vi "01_ui_main_loop.vi"() -> ()   [LabVIEW 2025]
uses:
  0417e9bc-26c0-40a3-857c-749a2451377f.vi
  040e489e-a473-4f93-bd06-0afa5652ce70.vi
  c6e3c1e2-0994-45fa-bff3-5cd5cb70e039.vi
  0bc7f4c2-ffb1-4822-9f64-357063f019c3.vi
  8b609e5e-a51d-4c52-8c18-d6a58a5b9e80.vi
  43d63275-3364-44ab-a9c8-6f7e055a0a8e.vi
  75836779-3642-44ab-91a1-288c14d5bff7.vi
  f856a27e-8979-4d67-ac65-7e3e0066168f.vi
  f6c46c24-e81c-4bed-970f-882e3bbfa33a.vi
  674b8dbc-10ac-464c-a410-8119d69976f5.vi
  efe7b7fb-95db-4648-be1d-36dd24965d64.vi
  a7921508-b016-4ad4-9c73-64ec30acdca8.vi
  2bf2835e-c011-4d5e-a055-403be64c671f.vi
  <vilib>/Utility/config.llb/Read Key (String).vi
  <vilib>/Utility/config.llb/Read Key (U32).vi
  <vilib>/Utility/config.llb/Read Key (Boolean).vi
  <vilib>/Utility/config.llb/Write Key (String).vi
  <vilib>/Utility/config.llb/Write Key (U32).vi
  <vilib>/Utility/config.llb/Write Key (Boolean).vi
  <vilib>/Utility/config.llb/NI_LVConfig.lvlib
panel:
  in  "color_picker_cursor_2":u32(colorbox)=16756736
  in  "color_picker_cursor_1":u32(colorbox)=11927752
  in  "sva_del_cal_file":bool
  in  "sva_cal_file":string(combo)
  in  "button_tcp_load_cal":bool caption="Connect"
  in  "button_tcp_smith_mode":bool caption="Connect"
  in  "button_tcp_s21_mode":bool caption="Connect"
  in  "button_tcp_s11_mode":bool caption="Connect"
  in  "button_tcp_vna_mode":bool caption="Connect"
  in  "show_plot_window":bool
  in  "button_save_s2p":bool caption="Save *.s2p"
  in  "button_tcp_connect":bool caption="Connect"
  in  "sva_port":u16=5025 caption="Port"
  in  "sva_ip":string="192.168.2.29" caption="IP"
  in  "stop":bool
  in  "button_auto_sweep":bool caption="Auto Sweep"
  in  "sweep_points":dbl caption="Points" min=0.0 step=1.0 format="%#_6f"
  in  "sweep_stop":dbl caption="Stop Frequency" min=0.0 step=1.0 format="%#_6f"
  in  "sweep_start":dbl caption="Start Frequency" min=0.0 step=1.0 format="%#_6f"
  in  "selector_serial_port":refnum<visa-resource-name>="COM1" caption="COM-Port"
  out "led_serial_connected":bool caption="Connected"
  in  "button_serial_connect":bool caption="Connect"
  in  "button_single_sweep":bool caption="Single Sweep"
  out "plot_smith_legend_curs_r":dbl caption="Cursor - R"
  out "plot_smith_legend_phase":dbl caption="Phase"
  out "plot_smith_legend_freq":string caption="Frequency"
  out "plot_smith_legend_jx":dbl caption="jX"
  out "plot_smith_legend_r":dbl caption="R"
  out "plot_smith":picture caption="Smith"
  out "filename":string caption="Recent File"
  in  "button_save_s1p":bool caption="Save *.s1p"
  in  "button_load_csv":bool caption="Load *.s1p 2"
  in  "button_load_sxp":bool caption="Load *.sxp"
  in  "show_smith_window":bool
  out "min_vswr_idx":i32
  in  "set_min_vswr_c2":bool
  in  "set_min_vswr_c1":bool
  out "min_vswr_freq":string caption="@ Frequency"
  out "min_vswr":dbl caption="Min. VSWR"
  out "min_frequency":string caption="Min. Frequency"
  out "points":dbl caption="Points"
  out "max_frequency":string caption="Max. Frequency"
  out "plot_smith_legend_curs_x":dbl caption="Cursor - jX"
  out "cursor_cp_1_prefix":string
  out "cursor_lp_1_prefix":string
  out "cursor_cs_1_prefix":string
  out "cursor_ls_1_prefix":string
  out "cursor_cp_2_prefix":string
  out "cursor_lp_2_prefix":string
  out "cursor_cs_2_prefix":string
  in  "lc_scale_settings":enum32{"autoscale", "fancy_scale", "zero_scale"}(radio)=enum."zero_scale"
  out "cursor_ls_2_prefix":string
  out "cursor_cp_2":dbl format="%#_6f"
  in  "color_picker_cp":u32(colorbox)=14468608
  out "cursor_cp_1":dbl format="%#_6f"
  in  "enable_plot_cp":bool=TRUE caption="S11 - Imaginary"
  out "cursor_lp_2":dbl format="%#_6f"
  in  "color_picker_lp":u32(colorbox)=39219
  out "cursor_lp_1":dbl format="%#_6f"
  in  "enable_plot_lp":bool caption="S11 - Imaginary"
  out "cursor_cs_2":dbl format="%#_6f"
  out "cursor_ls_2":dbl format="%#_6f"
  out "cursor_lc_freq_2":string caption="Frequenz"
  out "cursor_lc_wavel_2":dbl caption="Frequenz"
  out "cursor_lc_wavel_1":dbl caption="Frequenz"
  in  "color_picker_cs":u32(colorbox)=14423100
  in  "color_picker_ls":u32(colorbox)=26316
  out "cursor_lc_freq_1":string caption="Frequenz"
  out "cursor_cs_1":dbl format="%#_6f"
  out "cursor_ls_1":dbl format="%#_6f"
  in  "enable_plot_cs":bool caption="S11 - Imaginary"
  in  "enable_plot_ls":bool=TRUE caption="S11 - Real"
  out "plot_lc":cluster{"array type (2D Dbl)":dbl[], dbl[]}[](graph) caption="L+C (Serial) / Lp+Cp (Parallel)"
  out "cursor_z_2":dbl format="%#_6f"
  in  "color_picker_z":u32(colorbox)=13314815
  out "cursor_z_1":dbl format="%#_6f"
  in  "enable_plot_z":bool=TRUE caption="S11 - Imaginary"
  out "cursor_jxp_2":dbl format="%#_6f"
  in  "color_picker_jxp":u32(colorbox)=14468608
  out "cursor_jxp_1":dbl format="%#_6f"
  in  "enable_plot_jxp":bool caption="S11 - Imaginary"
  out "cursor_rp_2":dbl format="%#_6f"
  in  "color_picker_rp":u32(colorbox)=39219
  out "cursor_rp_1":dbl format="%#_6f"
  in  "enable_plot_rp":bool caption="S11 - Imaginary"
  out "cursor_jx_2":dbl format="%#_6f"
  out "cursor_r_2":dbl format="%#_6f"
  out "cursor_imag_2":dbl format="%#_6f"
  out "cursor_real_2":dbl format="%#_6f"
  out "cursor_r_jx_freq_2":string caption="Frequenz"
  out "cursor_r_jx_wavel_2":dbl caption="Frequenz"
  out "cursor_r_jx_wavel_1":dbl caption="Frequenz"
  out "cursor_real_imag_freq_2":string caption="Frequenz"
  out "cursor_real_imag_wavel_2":dbl caption="Frequenz"
  out "cursor_real_imag_wavel_1":dbl caption="Frequenz"
  out "cursor_log_phase_wavel_2":dbl caption="Frequenz"
  out "cursor_log_phase_wavel_1":dbl caption="Frequenz"
  in  "cursor_mode":bool=TRUE caption="Cursor Mode"
  out "cursor_vswr_2":dbl format="%#_6f"
  in  "color_picker_vswr":u32(colorbox)=39219
  out "cursor_vswr_1":dbl format="%#_6f"
  in  "enable_plot_vswr":bool=TRUE caption="S11 - VSWR"
  out "cursor_log_phase_freq_2":string caption="Frequenz"
  out "cursor_phase_2":dbl format="%#_6f"
  out "cursor_logmag_2":dbl format="%#_6f"
  in  "color_picker_jx":u32(colorbox)=14423100
  in  "color_picker_r":u32(colorbox)=26316
  out "cursor_r_jx_freq_1":string caption="Frequenz"
  out "cursor_jx_1":dbl format="%#_6f"
  out "cursor_r_1":dbl format="%#_6f"
  in  "enable_plot_jx":bool=TRUE caption="S11 - Imaginary"
  in  "enable_plot_r":bool=TRUE caption="S11 - Real"
  in  "color_picker_imag":u32(colorbox)=14423100
  in  "color_picker_real":u32(colorbox)=26316
  out "cursor_real_imag_freq_1":string caption="Frequenz"
  out "cursor_imag_1":dbl format="%#_6f"
  out "cursor_real_1":dbl format="%#_6f"
  in  "enable_plot_imag":bool=TRUE caption="S11 - Imaginary"
  in  "enable_plot_real":bool=TRUE caption="S11 - Real"
  out "plot_real_imag":cluster{"array type (2D Dbl)":dbl[], dbl[]}[](graph) caption="Real / Imaginary"
  in  "color_picker_phase":u32(colorbox)=14423100
  in  "color_picker_logmag":u32(colorbox)=26316
  out "cursor_log_phase_freq_1":string caption="Frequenz"
  out "cursor_phase_1":dbl format="%#_6f"
  out "cursor_logmag_1":dbl format="%#_6f"
  in  "rx_scale_settings":enum32{"autoscale", "fancy_scale"}(radio)=enum."fancy_scale"
  in  "enable_plot_phase":bool=TRUE caption="S11 - Phase"
  in  "enable_plot_logmag":bool=TRUE caption="S11 - Logmag"
  out "plot_rjx":cluster{"array type (2D Dbl)":dbl[], dbl[]}[](graph) caption="R+jX (Serial) / Rp+jXp (Parallel) / Z"
  out "plot_log_phase_vswr":cluster{"array type (2D Dbl)":dbl[], dbl[]}[](graph) caption="Logmag / Phase / VSWR"
  # "LabVNA - VNA/S-Parameter Software"
  # "by Robin Tönniges (DC7RT)"
  # "Hz"
  # "NanoVNA"
  # "Siglent SVA"
  # "Sweep"
  # "Trace Data"
  # "Load/Save"
  # "Cursor 1"
  # "Cursor 2"
  # "Frequency"
  # "Hz"
  # "Hz"
  # "Wavelength"
  # "m"
  # "m"
  # "Frequency"
  # "Hz"
  # "Hz"
  # "Wavelength"
  # "m"
  # "m"
  # "Hz"
  # "Frequency"
  # "Hz"
  # "Wavelength"
  # "m"
  # "m"
  # "Frequency [MHz]"
  # "Hz"
  # "Frequency"
  # "Hz"
  # "Wavelength"
  # "m"
  # "m"
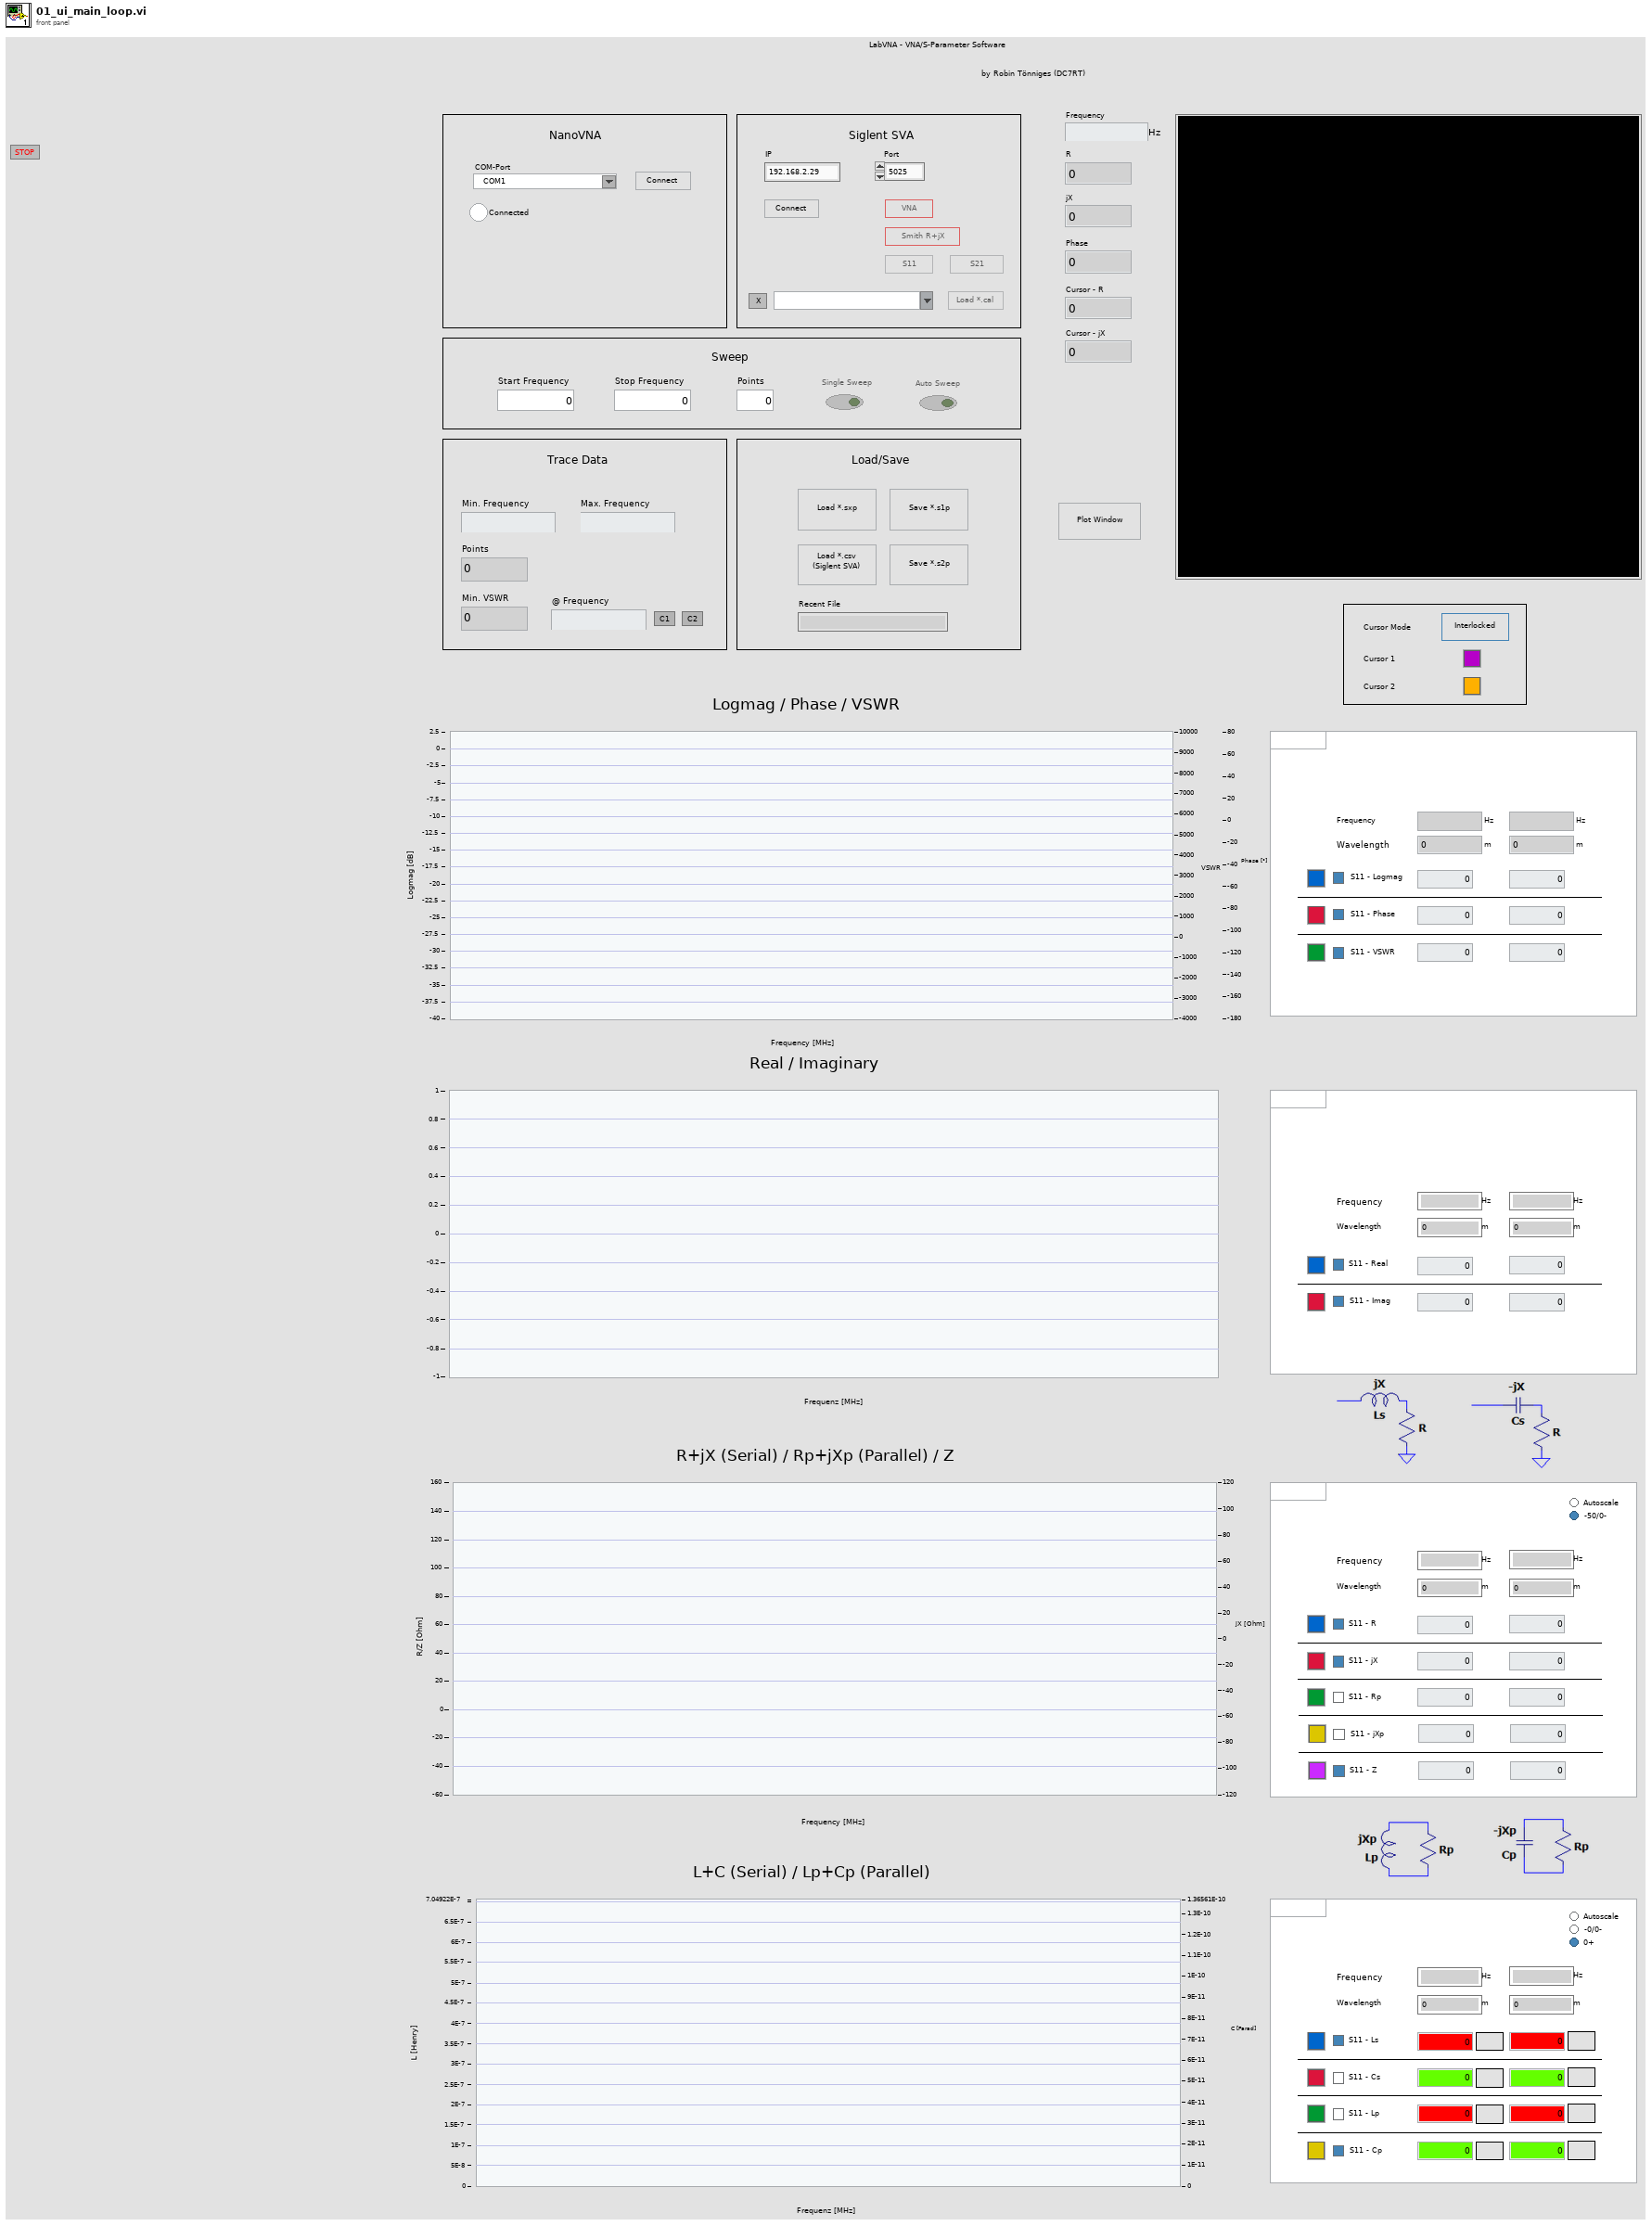
[diagram p1: front panel]
types:
  T1 = cluster{"button_serial_connect":bool, "button_auto_sweep":bool, "button_tcp_connect":bool}
  T2 = cluster{"button_load_sxp":bool, "button_load_csv":bool, "button_save_s1p":bool, "button_save_s2p":bool, "button_single_sweep":bool, "tcp_load_cal":bool}
  T3 = enum8{"Enabled", "Disabled", "Disabled and Grayed Out"}
  T4 = enum32{"Invalid", "Standard", "Closed", "Hidden", "Minimized", "Maximized"}
  T5 = cluster{"left":dbl, "top":dbl, "right":dbl, "bottom":dbl}
  T6 = cluster{"x":cluster{"a":dbl, "b":dbl, "log?":bool}, "y":cluster{"a":dbl, "b":dbl, "log?":bool}}
  T7 = typedef "NI_LVConfig.lvlib/Config Data RefNum.ctl" = refnum<k1>
  T8 = cluster{"button_load_sxp":bool, "button_load_csv":bool, "button_save_s1p":bool, "button_save_s2p":bool, "button_single_sweep":bool, "button_tcp_load_cal":bool}
  T9 = cluster{"mode":string, "s11_s21":string, "graph":string, "freq_range":cluster{"start_freq":string, "stop_freq":string}, "points":string}
  T10 = typedef "LVCursorListTypeDef.ctl" = cluster{"Name":string, "Color":u32, "Style":u8, "Point Style":u8, "Name Visible":bool, "Allow Drag":bool, "Cursor Mode":u32, "Plot":i32, "Index":i32, "Position":cluster{"X":dbl, "Y":dbl}, "X Scale":u32, "Y Scale":u32, "Watch Plots":i32[], "Watch All Plots":bool, "Plot Area":i32, "Label Offset":cluster{"X":dbl, "Y":dbl}}[]
  T11 = typedef "LVPoint32TypeDef.ctl" = cluster{"Horizontal":i32, "Vertical":i32}
  T12 = cluster{"frequency":dbl, "r":dbl, "jx":dbl, "phase":dbl}
  T13 = cluster{"cursor_data":dbl[], "frequency":string, "wavelength_m":dbl}
  T14 = cluster{"freq_array":dbl[], "data_array":dbl[]}[]
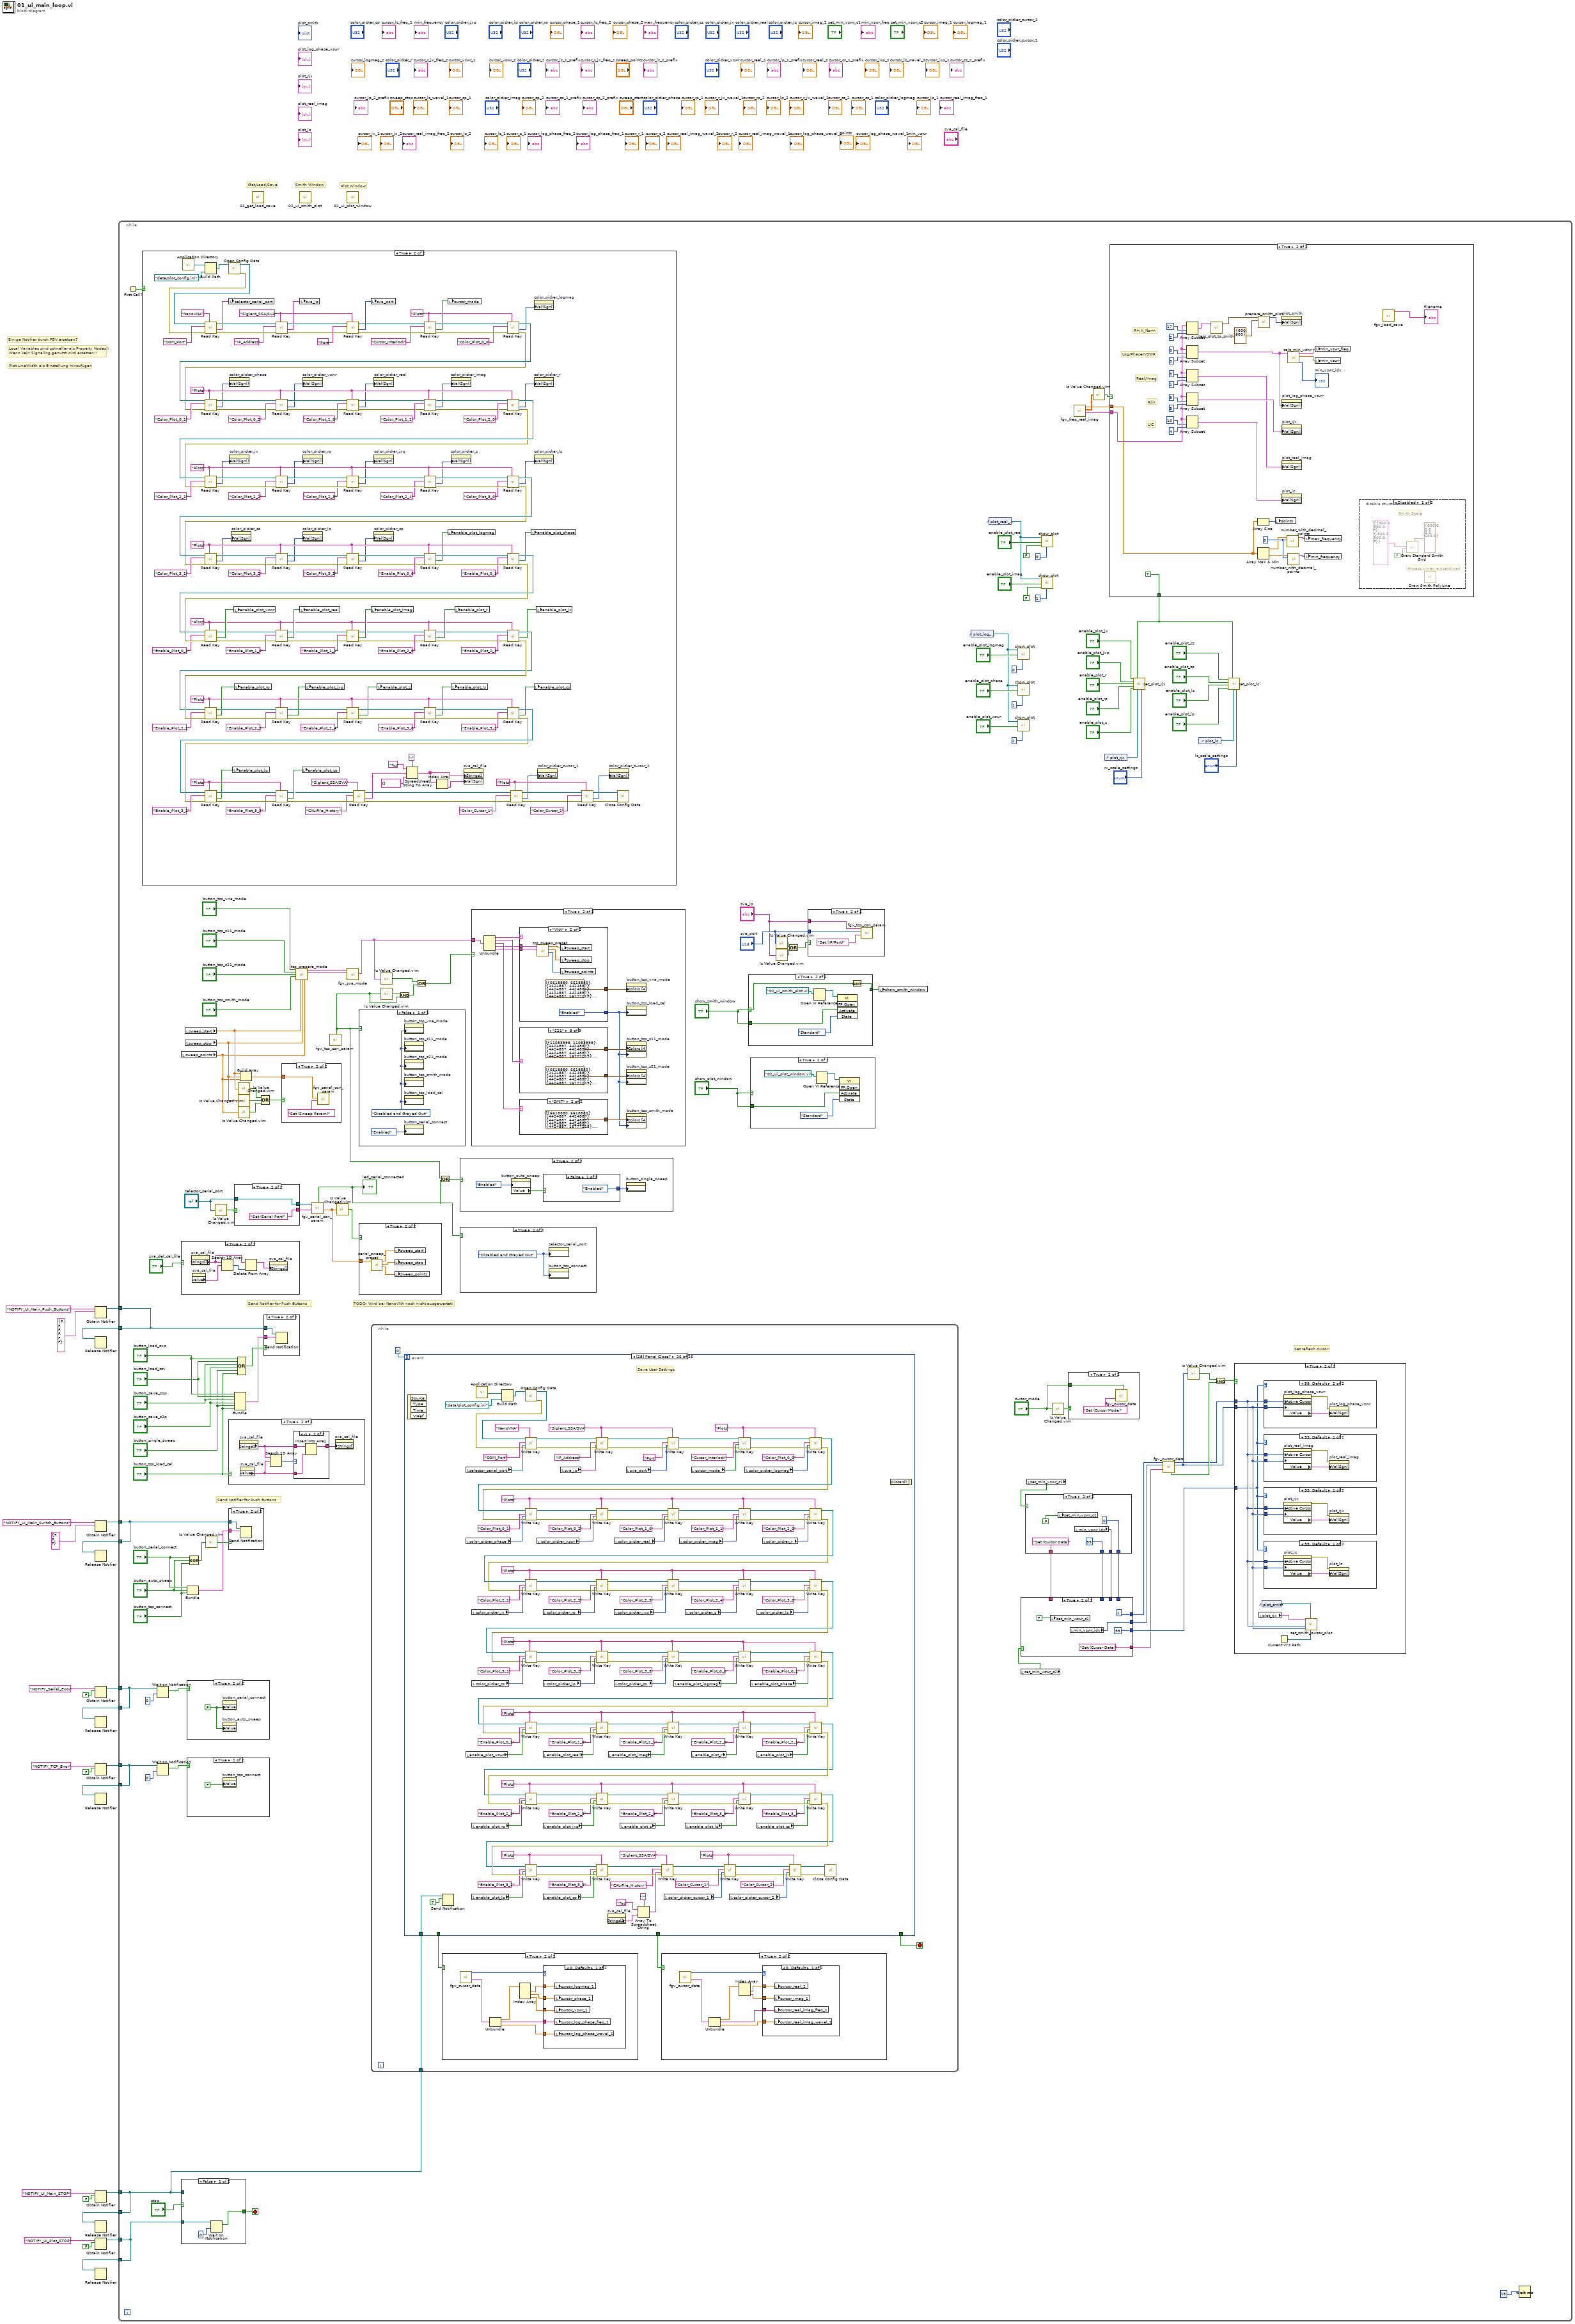
[diagram p0: block diagram]
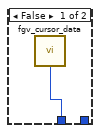
[diagram p9: hidden frame]
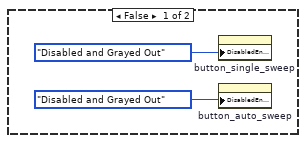
[diagram p11: hidden frame]
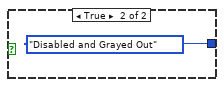
[diagram p12: hidden frame]
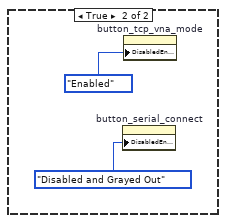
[diagram p16: hidden frame]
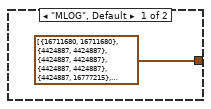
[diagram p18: hidden frame]
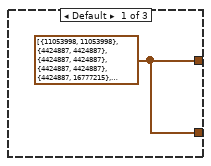
[diagram p19: hidden frame]
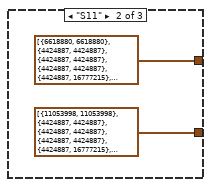
[diagram p20: hidden frame]
diagram:
  # "Plot LineWidth als Einstellung hinzufügen"
  # "Local Variables sind schneller als Property Nodes!!\nWenn kein Signaling genutzt wird ersetzen!!"
  # "Einige Notifier durch FGV ersetzen?"
  # "Plot Window"
  # "Get/Load/Save"
  # "Smith WIndow"
  n1 = Obtain Notifier(name (unnamed)="NOTIFY_UI_Main_Push_Buttons", notification data type=T2 {"button_load_sxp"=FALSE, "button_load_csv"=FALSE, "button_save_s1p"=FALSE, "button_save_s2p"=FALSE, "button_single_sweep"=FALSE, "tcp_load_cal"=FALSE} ("output cluster")) -> (notifier out=w23:refnum<notifier>)  [unwired: 2 in, 2 out]
  n2 = Obtain Notifier(name (unnamed)="NOTIFY_UI_Main_Switch_Buttons", notification data type=T1 {"button_serial_connect"=FALSE, "button_auto_sweep"=FALSE, "button_tcp_connect"=FALSE} ("output cluster")) -> (notifier out=w12:refnum<notifier>)  [unwired: 2 in, 2 out]
  n3 = Obtain Notifier(name (unnamed)="NOTIFY_Serial_Error", notification data type=FALSE) -> (notifier out=w15:refnum<notifier>)  [unwired: 2 in, 2 out]
  n4 = Obtain Notifier(name (unnamed)="NOTIFY_TCP_Error", notification data type=FALSE) -> (notifier out=w3:refnum<notifier>)  [unwired: 2 in, 2 out]
  n5 = Obtain Notifier(name (unnamed)="NOTIFY_UI_Main_STOP", notification data type=FALSE) -> (notifier out=w20:refnum<notifier>)  [unwired: 2 in, 2 out]
  n6 = Obtain Notifier(name (unnamed)="NOTIFY_UI_Plot_STOP", notification data type=FALSE) -> (notifier out=w6:refnum<notifier>)  [unwired: 2 in, 2 out]
  n7 = while {
    tunnel: w23 -> [w107]
    tunnel: [w107] -> w22
    tunnel: w20 -> [w84]
    tunnel: [w84] -> w21
    tunnel: w15 -> [w99]
    tunnel: [w99] -> w14
    tunnel: w12 -> [w96]
    tunnel: [w96] -> w13
    tunnel: [w73] -> w7
    tunnel: w6 -> [w73]
    tunnel: w3 -> [w66]
    tunnel: [w66] -> w4
    stop <- w100 stop-if-true
    # "Set refresh cursor"
    # "TODO: Wird bei NanoVNA noch nicht ausgewertet!"
    # "Send Notifier for Push Buttons"
    # "Send Notifier for Push Buttons"
    n8 = First Call?() -> (First Call?: T/F=w74:bool)
    n9 = case shown="True" w74 {
      frame False {
      }
      frame True {
        w251 = "Plots" ("section")
        w281 = "Plots" ("section")
        w272 = "Plots" ("section")
        w302 = "Plots" ("section")
        w271 = "Plots" ("section")
        w355 = "Plots" ("section")
        w356 = "Plots" ("section")
        w369 = "Plots" ("section")
        w370 = "Siglent_SSA/SVA" ("section")
        n10 = call <vilib>:"Application Directory.vi"() -> ("Application Directory"=w266:path)
        n11 = Build Path(base path=w266, name or relative path=path "data/plot_config.ini") -> (appended path=w270:path)
        n12 = call <vilib>:"Open Config Data.vi"("configuration file path"=w270) -> ("error out"=w268:errorcluster, "refnum"=w267:T7)  [unwired: 8 in, 1 out]
        n13 = call-poly <vilib>:"Read Key.vi"("section"="NanoVNA", "error in (no error)"=w268, "key"="COM_Port", "refnum"=w267) -> ("error out"=w386:errorcluster, "value"=w389:string, "refnum out"=w387:T7)  [unwired: 4 in, 1 out]
        n14 = local write "selector_serial_port"(w389) -> ()
        n15 = call-poly <vilib>:"Read Key.vi"("section"=w370, "error in (no error)"=w386, "key"="IP_Address", "refnum"=w387) -> ("error out"=w382:errorcluster, "value"=w385:string, "refnum out"=w383:T7)  [unwired: 4 in, 1 out]
        n16 = local write "sva_ip"(w385) -> ()
        n17 = call-poly <vilib>:"Read Key.vi"("section"=w370, "error in (no error)"=w382, "key"="Port", "refnum"=w383) -> ("error out"=w378:errorcluster, "value"=w381:u32, "refnum out"=w379:T7)  [unwired: 4 in, 1 out]
        n18 = local write "sva_port"(w381) -> ()
        n19 = call-poly <vilib>:"Read Key.vi"("section"=w369, "error in (no error)"=w378, "key"="Cursor_Interlock", "refnum"=w379) -> ("error out"=w374:errorcluster, "value"=w377:bool, "refnum out"=w375:T7)  [unwired: 4 in, 1 out]
        n20 = local write "cursor_mode"(w377) -> ()
        n21 = call-poly <vilib>:"Read Key.vi"("section"=w369, "error in (no error)"=w374, "key"="Color_Plot_0_0", "refnum"=w375) -> ("error out"=w371:errorcluster, "value"=w246:u32, "refnum out"=w372:T7)  [unwired: 4 in, 1 out]
        n22 = call-poly <vilib>:"Read Key.vi"("section"=w356, "error in (no error)"=w371, "key"="Color_Plot_0_1", "refnum"=w372) -> ("error out"=w366:errorcluster, "value"=w245:u32, "refnum out"=w367:T7)  [unwired: 4 in, 1 out]
        n23 = property on="color_picker_phase" class="ColBox"("Val(Sgnl)"=w245) -> ()  [unwired: 2 in, 2 out]
        n24 = call-poly <vilib>:"Read Key.vi"("section"=w356, "error in (no error)"=w366, "key"="Color_Plot_0_2", "refnum"=w367) -> ("error out"=w363:errorcluster, "value"=w244:u32, "refnum out"=w364:T7)  [unwired: 4 in, 1 out]
        n25 = property on="color_picker_vswr" class="ColBox"("Val(Sgnl)"=w244) -> ()  [unwired: 2 in, 2 out]
        n26 = call-poly <vilib>:"Read Key.vi"("section"=w356, "error in (no error)"=w363, "key"="Color_Plot_1_0", "refnum"=w364) -> ("error out"=w360:errorcluster, "value"=w243:u32, "refnum out"=w361:T7)  [unwired: 4 in, 1 out]
        n27 = property on="color_picker_real" class="ColBox"("Val(Sgnl)"=w243) -> ()  [unwired: 2 in, 2 out]
        n28 = call-poly <vilib>:"Read Key.vi"("section"=w356, "error in (no error)"=w360, "key"="Color_Plot_1_1", "refnum"=w361) -> ("error out"=w357:errorcluster, "value"=w242:u32, "refnum out"=w358:T7)  [unwired: 4 in, 1 out]
        n29 = property on="color_picker_imag" class="ColBox"("Val(Sgnl)"=w242) -> ()  [unwired: 2 in, 2 out]
        n30 = call-poly <vilib>:"Read Key.vi"("section"=w356, "error in (no error)"=w357, "key"="Color_Plot_2_0", "refnum"=w358) -> ("error out"=w340:errorcluster, "value"=w241:u32, "refnum out"=w341:T7)  [unwired: 4 in, 1 out]
        n31 = call-poly <vilib>:"Read Key.vi"("section"=w355, "error in (no error)"=w340, "key"="Color_Plot_2_1", "refnum"=w341) -> ("error out"=w345:errorcluster, "value"=w240:u32, "refnum out"=w344:T7)  [unwired: 4 in, 1 out]
        n32 = property on="color_picker_jx" class="ColBox"("Val(Sgnl)"=w240) -> ()  [unwired: 2 in, 2 out]
        n33 = call-poly <vilib>:"Read Key.vi"("section"=w355, "error in (no error)"=w345, "key"="Color_Plot_2_2", "refnum"=w344) -> ("error out"=w348:errorcluster, "value"=w239:u32, "refnum out"=w347:T7)  [unwired: 4 in, 1 out]
        n34 = property on="color_picker_rp" class="ColBox"("Val(Sgnl)"=w239) -> ()  [unwired: 2 in, 2 out]
        n35 = call-poly <vilib>:"Read Key.vi"("section"=w355, "error in (no error)"=w348, "key"="Color_Plot_2_3", "refnum"=w347) -> ("error out"=w351:errorcluster, "value"=w238:u32, "refnum out"=w350:T7)  [unwired: 4 in, 1 out]
        n36 = property on="color_picker_jxp" class="ColBox"("Val(Sgnl)"=w238) -> ()  [unwired: 2 in, 2 out]
        n37 = call-poly <vilib>:"Read Key.vi"("section"=w355, "error in (no error)"=w351, "key"="Color_Plot_2_4", "refnum"=w350) -> ("error out"=w354:errorcluster, "value"=w237:u32, "refnum out"=w353:T7)  [unwired: 4 in, 1 out]
        n38 = property on="color_picker_z" class="ColBox"("Val(Sgnl)"=w237) -> ()  [unwired: 2 in, 2 out]
        n39 = call-poly <vilib>:"Read Key.vi"("section"=w355, "error in (no error)"=w354, "key"="Color_Plot_3_0", "refnum"=w353) -> ("error out"=w331:errorcluster, "value"=w236:u32, "refnum out"=w332:T7)  [unwired: 4 in, 1 out]
        n40 = call-poly <vilib>:"Read Key.vi"("section"=w271, "error in (no error)"=w331, "key"="Color_Plot_3_1", "refnum"=w332) -> ("error out"=w336:errorcluster, "value"=w235:u32, "refnum out"=w337:T7)  [unwired: 4 in, 1 out]
        n41 = property on="color_picker_cs" class="ColBox"("Val(Sgnl)"=w235) -> ()  [unwired: 2 in, 2 out]
        n42 = call-poly <vilib>:"Read Key.vi"("section"=w271, "error in (no error)"=w336, "key"="Color_Plot_3_2", "refnum"=w337) -> ("error out"=w333:errorcluster, "value"=w234:u32, "refnum out"=w334:T7)  [unwired: 4 in, 1 out]
        n43 = property on="color_picker_lp" class="ColBox"("Val(Sgnl)"=w234) -> ()  [unwired: 2 in, 2 out]
        n44 = call-poly <vilib>:"Read Key.vi"("section"=w271, "error in (no error)"=w333, "key"="Color_Plot_3_3", "refnum"=w334) -> ("error out"=w295:errorcluster, "value"=w233:u32, "refnum out"=w294:T7)  [unwired: 4 in, 1 out]
        n45 = property on="color_picker_cp" class="ColBox"("Val(Sgnl)"=w233) -> ()  [unwired: 2 in, 2 out]
        n46 = call-poly <vilib>:"Read Key.vi"("section"=w271, "error in (no error)"=w295, "key"="Enable_Plot_0_0", "refnum"=w294) -> ("error out"=w300:errorcluster, "value"=w297:bool, "refnum out"=w299:T7)  [unwired: 4 in, 1 out]
        n47 = local write "enable_plot_logmag"(w297) -> ()
        n48 = call-poly <vilib>:"Read Key.vi"("section"=w271, "error in (no error)"=w300, "key"="Enable_Plot_0_1", "refnum"=w299) -> ("error out"=w322:errorcluster, "value"=w301:bool, "refnum out"=w321:T7)  [unwired: 4 in, 1 out]
        n49 = call-poly <vilib>:"Read Key.vi"("section"=w302, "error in (no error)"=w322, "key"="Enable_Plot_0_2", "refnum"=w321) -> ("error out"=w315:errorcluster, "value"=w319:bool, "refnum out"=w316:T7)  [unwired: 4 in, 1 out]
        n50 = local write "enable_plot_vswr"(w319) -> ()
        n51 = call-poly <vilib>:"Read Key.vi"("section"=w302, "error in (no error)"=w315, "key"="Enable_Plot_1_0", "refnum"=w316) -> ("error out"=w311:errorcluster, "value"=w318:bool, "refnum out"=w312:T7)  [unwired: 4 in, 1 out]
        n52 = local write "enable_plot_real"(w318) -> ()
        n53 = call-poly <vilib>:"Read Key.vi"("section"=w302, "error in (no error)"=w311, "key"="Enable_Plot_1_1", "refnum"=w312) -> ("error out"=w307:errorcluster, "value"=w313:bool, "refnum out"=w309:T7)  [unwired: 4 in, 1 out]
        n54 = local write "enable_plot_imag"(w313) -> ()
        n55 = call-poly <vilib>:"Read Key.vi"("section"=w302, "error in (no error)"=w307, "key"="Enable_Plot_2_0", "refnum"=w309) -> ("error out"=w304:errorcluster, "value"=w308:bool, "refnum out"=w305:T7)  [unwired: 4 in, 1 out]
        n56 = local write "enable_plot_r"(w308) -> ()
        n57 = call-poly <vilib>:"Read Key.vi"("section"=w302, "error in (no error)"=w304, "key"="Enable_Plot_2_1", "refnum"=w305) -> ("error out"=w330:errorcluster, "value"=w303:bool, "refnum out"=w329:T7)  [unwired: 4 in, 1 out]
        n58 = call-poly <vilib>:"Read Key.vi"("section"=w272, "error in (no error)"=w330, "key"="Enable_Plot_2_2", "refnum"=w329) -> ("error out"=w328:errorcluster, "value"=w324:bool, "refnum out"=w327:T7)  [unwired: 4 in, 1 out]
        n59 = local write "enable_plot_rp"(w324) -> ()
        n60 = call-poly <vilib>:"Read Key.vi"("section"=w272, "error in (no error)"=w328, "key"="Enable_Plot_2_3", "refnum"=w327) -> ("error out"=w283:errorcluster, "value"=w325:bool, "refnum out"=w282:T7)  [unwired: 4 in, 1 out]
        n61 = local write "enable_plot_jxp"(w325) -> ()
        n62 = call-poly <vilib>:"Read Key.vi"("section"=w272, "error in (no error)"=w283, "key"="Enable_Plot_2_4", "refnum"=w282) -> ("error out"=w289:errorcluster, "value"=w285:bool, "refnum out"=w287:T7)  [unwired: 4 in, 1 out]
        n63 = local write "enable_plot_z"(w285) -> ()
        n64 = call-poly <vilib>:"Read Key.vi"("section"=w272, "error in (no error)"=w289, "key"="Enable_Plot_3_0", "refnum"=w287) -> ("error out"=w292:errorcluster, "value"=w288:bool, "refnum out"=w291:T7)  [unwired: 4 in, 1 out]
        n65 = local write "enable_plot_ls"(w288) -> ()
        n66 = call-poly <vilib>:"Read Key.vi"("section"=w272, "error in (no error)"=w292, "key"="Enable_Plot_3_1", "refnum"=w291) -> ("error out"=w273:errorcluster, "value"=w293:bool, "refnum out"=w274:T7)  [unwired: 4 in, 1 out]
        n67 = call-poly <vilib>:"Read Key.vi"("section"=w281, "error in (no error)"=w273, "key"="Enable_Plot_3_2", "refnum"=w274) -> ("error out"=w280:errorcluster, "value"=w276:bool, "refnum out"=w279:T7)  [unwired: 4 in, 1 out]
        n68 = local write "enable_plot_lp"(w276) -> ()
        n69 = call-poly <vilib>:"Read Key.vi"("section"=w281, "error in (no error)"=w280, "key"="Enable_Plot_3_3", "refnum"=w279) -> ("error out"=w262:errorcluster, "value"=w277:bool, "refnum out"=w263:T7)  [unwired: 4 in, 1 out]
        n70 = local write "enable_plot_cp"(w277) -> ()
        n71 = call-poly <vilib>:"Read Key.vi"("section"="Siglent_SSA/SVA", "error in (no error)"=w262, "key"="CAL-File_History", "refnum"=w263) -> ("error out"=w253:errorcluster, "value"=w265:string, "refnum out"=w254:T7)  [unwired: 4 in, 1 out]
        n72 = Spreadsheet String To Array(delimiter (Tab)=";", format string="%s", spreadsheet string=w265, array type (2D Dbl)=string[] []) -> (array=w257:string[])
        n73 = Index Array(array=w257) -> (element=w256:string)  [unwired: 1 in]
        n74 = property on="sva_cal_file" class="CmbBox"("Strings[]"=w257, "Val(Sgnl)"=w256) -> ()  [unwired: 2 in, 2 out]
        n75 = call-poly <vilib>:"Read Key.vi"("section"=w251, "error in (no error)"=w253, "key"="Color_Cursor_1", "refnum"=w254) -> ("error out"=w247:errorcluster, "value"=w232:u32, "refnum out"=w248:T7)  [unwired: 4 in, 1 out]
        n76 = local write "enable_plot_phase"(w301) -> ()
        n77 = property on="color_picker_logmag" class="ColBox"("Val(Sgnl)"=w246) -> ()  [unwired: 2 in, 2 out]
        n78 = property on="color_picker_r" class="ColBox"("Val(Sgnl)"=w241) -> ()  [unwired: 2 in, 2 out]
        n79 = property on="color_picker_ls" class="ColBox"("Val(Sgnl)"=w236) -> ()  [unwired: 2 in, 2 out]
        n80 = local write "enable_plot_cs"(w293) -> ()
        n81 = local write "enable_plot_jx"(w303) -> ()
        n82 = property on="color_picker_cursor_1" class="ColBox"("Val(Sgnl)"=w232) -> ()  [unwired: 2 in, 2 out]
        n83 = call-poly <vilib>:"Read Key.vi"("section"=w251, "error in (no error)"=w247, "key"="Color_Cursor_2", "refnum"=w248) -> ("error out"=w249:errorcluster, "value"=w231:u32, "refnum out"=w250:T7)  [unwired: 4 in, 1 out]
        n84 = property on="color_picker_cursor_2" class="ColBox"("Val(Sgnl)"=w231) -> ()  [unwired: 2 in, 2 out]
        n85 = call <vilib>:"Close Config Data.vi"("error in (no error)"=w249, "refnum"=w250) -> ()  [unwired: 8 in, 2 out]
      }
    }
    n86 = Wait on Notification(notifier=w99, timeout in ms (-1)=0) -> (notification=w97:bool)  [unwired: 2 in, 3 out]
    n87 = Wait on Notification(notifier=w66, timeout in ms (-1)=0) -> (notification=w68:bool)  [unwired: 2 in, 3 out]
    n88 = case shown="True" "sva_del_cal_file" {
      frame False {
      }
      frame True {
        n89 = property on="sva_cal_file" class="CmbBox"() -> ("Strings[]"=w188:string[])  [unwired: 2 in, 2 out]
        n90 = property on="sva_cal_file" class="CmbBox"() -> ("Value"=w190:string)  [unwired: 2 in, 2 out]
        n91 = Search 1D Array(1D array=w188, element=w190) -> (index of element=w189:i32)  [unwired: 1 in]
        n92 = Delete From Array(array=w188, index=w189) -> (array with subset deleted=w187:string[])  [unwired: 1 in, 1 out]
        n93 = property on="sva_cal_file" class="CmbBox"("Strings[]"=w187) -> ()  [unwired: 2 in, 2 out]
      }
    }
    n94 = case shown="False" "stop" {
      selector: "stop" -> [_ w406]
      tunnel: w84 -> [_ w407]
      tunnel: [w403 FALSE] -> w100
      tunnel: w73 -> [w402 _]
      frame False {
        n95 = Wait on Notification(notifier=w402, timeout in ms (-1)=0) -> (notification=w403:bool)  [unwired: 2 in, 3 out]
      }
      frame True {
        n96 = Send Notification(notification=w406, notifier=w407) -> ()  [unwired: 1 in, 2 out]
      }
    }
    n97 = local read "sweep_points"() -> (w43:dbl)
    n98 = local read "sweep_start"() -> (w45:dbl)
    n99 = local read "sweep_stop"() -> (w44:dbl)
    n100 = Bundle("button_serial_connect"="button_serial_connect", "button_auto_sweep"="button_auto_sweep", "button_tcp_connect"="button_tcp_connect") -> (w69:T1)  [unwired: 1 in]
    n101 = case shown="True" w97 {
      frame False {
      }
      frame True {
        w401 = FALSE
        n102 = property on="button_serial_connect" class="Bool (strict)"("Value"=w401) -> ()  [unwired: 2 in, 2 out]
        n103 = property on="button_auto_sweep" class="Bool (strict)"("Value"=w401) -> ()  [unwired: 2 in, 2 out]
      }
    }
    n104 = case shown="True" w68 {
      frame False {
      }
      frame True {
        n105 = property on="button_tcp_connect" class="Bool (strict)"("Value"=FALSE) -> ()  [unwired: 2 in, 2 out]
      }
    }
    n106 = Compound Arithmetic op=XOR("button_serial_connect", "button_auto_sweep", "button_tcp_connect") -> (w91:bool)
    n107 = call "Is Value Changed.vim"("value"=w91) -> ("changed or first call?"=w92:bool)
    n108 = call "Is Value Changed.vim"("value"="selector_serial_port") -> ("changed or first call?"=w136:bool)
    n109 = case shown="True" "button_tcp_load_cal" {
      frame False {
      }
      frame True {
        n110 = property on="sva_cal_file" class="CmbBox"() -> ("Strings[]"=w193:string[])  [unwired: 2 in, 2 out]
        n111 = property on="sva_cal_file" class="CmbBox"() -> ("Value"=w192:string)  [unwired: 2 in, 2 out]
        n112 = Search 1D Array(1D array=w193, element=w192) -> (index of element=w194:i32)  [unwired: 1 in]
        n113 = case shown="-1" w194 {
          tunnel: w193 -> [w195 w198]
          tunnel: w192 -> [_ w197]
          tunnel: [w195 w196] -> w191
          frame 0, Default {
          }
          frame -1 {
            n114 = Insert Into Array(array=w198, new element=w197) -> (w196:string[])  [unwired: 1 in]
          }
        }
        n115 = property on="sva_cal_file" class="CmbBox"("Strings[]"=w191) -> ()  [unwired: 2 in, 2 out]
      }
    }
    n116 = case shown="True" w92 {
      tunnel: w96 -> [_ w400]
      tunnel: w69 -> [_ w399]
      frame False {
      }
      frame True {
        n117 = Send Notification(notification=w399, notifier=w400) -> ()  [unwired: 1 in, 2 out]
      }
    }
    n118 = case shown="True" w136 {
      tunnel: "selector_serial_port" -> [_ w417]
      tunnel: ["Get" ("mode") "Set (Serial Port)" ("mode")] -> w75
      tunnel: [_ w417] -> w76
      frame False {
      }
      frame True {
      }
    }
    n119 = Bundle("button_load_sxp"="button_load_sxp", "button_load_csv"="button_load_csv", "button_save_s1p"="button_save_s1p", "button_save_s2p"="button_save_s2p", "button_single_sweep"="button_single_sweep", "button_tcp_load_cal"="button_tcp_load_cal") -> (w79:T8)  [unwired: 1 in]
    n120 = Compound Arithmetic op=OR("button_load_sxp", "button_load_csv", "button_save_s1p", "button_save_s2p", "button_single_sweep", "button_tcp_load_cal") -> (w102:bool)
    n121 = call "Is Value Changed.vim"("value"=w45) -> ("changed or first call?"=w48:bool)
    n122 = call "Is Value Changed.vim"("value"=w44) -> ("changed or first call?"=w49:bool)
    n123 = call "Is Value Changed.vim"("value"=w43) -> ("changed or first call?"=w47:bool)
    n124 = Build Array(w45, w44, w43) -> (w42:dbl[])
    n125 = Compound Arithmetic op=OR(w48, w49, w47) -> (w46:bool)
    n126 = case shown="True" w102 {
      tunnel: w107 -> [_ w409]
      tunnel: w79 -> [_ w408]
      frame False {
      }
      frame True {
        n127 = Send Notification(notification=w408, notifier=w409) -> ()  [unwired: 1 in, 2 out]
      }
    }
    n128 = case shown="True" w46 {
      tunnel: w42 -> [_ w178]
      frame False {
      }
      frame True {
        n129 = call "fgv_serial_con_param.vi"("mode"="Set (Sweep Param)", "sweep_param_set"=w178) -> ()  [unwired: 5 in, 5 out]
      }
    }
    n130 = call "tcp_prepare_mode.vi"("button_tcp_vna_mode"="button_tcp_vna_mode", "button_tcp_s11_mode"="button_tcp_s11_mode", "button_tcp_s21_mode"="button_tcp_s21_mode", "button_tcp_smith_mode"="button_tcp_smith_mode", "sweep_start"=w45, "sweep_stop"=w44, "sweep_points"=w43) -> ("mode"=w58:string, "data_out"=w57:T9)  [unwired: 7 in]
    n131 = call "fgv_serial_con_param.vi"("mode"=w75, "serial_port_set"=w76) -> ("sweep_param_get"=w77:dbl[], "serial_conn_get"=w51:bool)  [unwired: 5 in, 3 out]
    "led_serial_connected" <- w51
    n132 = call "fgv_tcp_con_param.vi"() -> ("tcp_connected_get"=w50:bool)  [unwired: 8 in, 3 out]
    n133 = call "Is Value Changed.vim"("value"=w77) -> ("changed or first call?"=w134:bool)
    n134 = call "fgv_sva_mode.vi"("data_in"=w57, "mode"=w58) -> ("data_out"=w65:T9)  [unwired: 7 in, 2 out]
    n135 = case shown="False" w50 {
      frame False {
        w200 = T3."Disabled and Grayed Out" ("DisabledEnum")
        n136 = property on="button_tcp_vna_mode" class="Bool"("DisabledEnum"=w200) -> ()  [unwired: 2 in, 2 out]
        n137 = property on="button_tcp_s11_mode" class="Bool"("DisabledEnum"=w200) -> ()  [unwired: 2 in, 2 out]
        n138 = property on="button_tcp_s21_mode" class="Bool"("DisabledEnum"=w200) -> ()  [unwired: 2 in, 2 out]
        n139 = property on="button_tcp_smith_mode" class="Bool"("DisabledEnum"=w200) -> ()  [unwired: 2 in, 2 out]
        n140 = property on="button_tcp_load_cal" class="Bool"("DisabledEnum"=w200) -> ()  [unwired: 2 in, 2 out]
        n141 = property on="button_serial_connect" class="Bool (strict)"("DisabledEnum"=T3."Enabled" ("Disabled")) -> ()  [unwired: 2 in, 2 out]
      }
      frame True {
        n142 = property on="button_serial_connect" class="Bool (strict)"("DisabledEnum"=T3."Disabled and Grayed Out" ("Disabled")) -> ()  [unwired: 2 in, 2 out]
        n143 = property on="button_tcp_vna_mode" class="Bool"("DisabledEnum"=T3."Enabled") -> ()  [unwired: 2 in, 2 out]
      }
    }
    n144 = case shown="True" w134 {
      tunnel: w77 -> [_ w413]
      frame False {
      }
      frame True {
        n145 = call "serial_sweep_preset.vi"("sweep_data"=w413) -> ("sweep_points"=w412:dbl, "sweep_stop"=w411:dbl, "sweep_start"=w410:dbl)  [unwired: 8 in]
        n146 = local write "sweep_start"(w410) -> ()
        n147 = local write "sweep_stop"(w411) -> ()
        n148 = local write "sweep_points"(w412) -> ()
      }
    }
    n149 = while {
      tunnel: w84 -> [w428]
      stop <- w429 stop-if-true
      n150 = event shown="[25] Panel Close?" {
        selector: _ -> [_ _ _ _ _ _ _ _ _ _ _ _ _ _ _ _ _ _ _ _ _ _ _ _ _ _]
        dyn-events: _ -> [_ _ _ _ _ _ _ _ _ _ _ _ _ _ _ _ _ _ _ _ _ _ _ _ _ _]
        timeout: 0 -> [_ _ _ _ _ _ _ _ _ _ _ _ _ _ _ _ _ _ _ _ _ _ _ _ _ _]
        tunnel: [_ _ _ _ _ _ _ _ _ _ _ _ _ _ _ _ _ _ _ _ _ _ _ _ TRUE _] -> w429
        tunnel: w428 -> [_ _ _ _ _ _ _ _ _ _ _ _ _ _ _ _ _ _ _ _ _ _ _ _ _ w980]
        tunnel: [_ _ TRUE _ _ _ _ _ _ _ _ _ _ _ _ _ _ _ _ _ _ _ _ _ _ _] -> w427
        tunnel: [_ _ _ _ _ _ _ TRUE _ _ _ _ _ _ _ _ _ _ _ _ _ _ _ _ _ _] -> w426
        event "color_picker_cursor_1": Value Change {
          w472 = u32 0 ("Active Plot")
          n151 = event-data() -> ("NewVal"=w465:u32)  [unwired: 1 in, 5 out]
          n152 = Bundle("NewVal"=w465, "NewVal"=w465) -> (w466:cluster{"NewVal":u32, "NewVal":u32})  [unwired: 1 in]
          n153 = property on="plot_real_imag" class="XYGraph (strict)"("Active Cursor"=w472, "Cursor.Cursor Color"=w465) -> ()  [unwired: 2 in, 2 out]
          n154 = property on="plot_rjx" class="XYGraph (strict)"("Active Cursor"=w472, "Cursor.Cursor Color"=w465) -> ()  [unwired: 2 in, 2 out]
          n155 = property on="plot_lc" class="XYGraph (strict)"("Active Cursor"=w472, "Cursor.Cursor Color"=w465) -> ()  [unwired: 2 in, 2 out]
          n156 = property on="plot_log_phase_vswr" class="XYGraph (strict)"("Active Cursor"=w472, "Cursor.Cursor Color"=w465) -> ()  [unwired: 2 in, 2 out]
          n157 = property class="VI"() -> (error out=w470:errorcluster, "Front Panel"=w469:refnum<vi>)  [unwired: 2 in, 1 out]
          n158 = call "fgv_cursor_data.vi"("cursor_color_set"=w466, "mode"="Set (Cursor 0 Color)") -> ()  [unwired: 7 in, 7 out]
          n159 = property class="Pnl"(reference=w469, error in=w470) -> ("Decorations[]"=w468:refnum<vi>[])  [unwired: 2 out]
          n160 = Index Array(array=w468, index=0) -> (element=w471:refnum<vi>)
          n161 = property class="Decor"(reference=w471, "BG Color"=w465, "FG Color"=w465) -> ()  [unwired: 1 in, 2 out]
        }
        event "color_picker_cursor_2": Value Change {
          w481 = u32 1 ("Active Plot")
          n162 = event-data() -> ("NewVal"=w473:u32)  [unwired: 1 in, 5 out]
          n163 = Bundle("NewVal"=w473, "NewVal"=w473) -> (w475:cluster{"NewVal":u32, "NewVal":u32})  [unwired: 1 in]
          n164 = property on="plot_real_imag" class="XYGraph (strict)"("Active Cursor"=w481, "Cursor.Cursor Color"=w473) -> ()  [unwired: 2 in, 2 out]
          n165 = property on="plot_rjx" class="XYGraph (strict)"("Active Cursor"=w481, "Cursor.Cursor Color"=w473) -> ()  [unwired: 2 in, 2 out]
          n166 = property on="plot_lc" class="XYGraph (strict)"("Active Cursor"=w481, "Cursor.Cursor Color"=w473) -> ()  [unwired: 2 in, 2 out]
          n167 = property on="plot_log_phase_vswr" class="XYGraph (strict)"("Active Cursor"=w481, "Cursor.Cursor Color"=w473) -> ()  [unwired: 2 in, 2 out]
          n168 = property class="VI"() -> (error out=w479:errorcluster, "Front Panel"=w478:refnum<vi>)  [unwired: 2 in, 1 out]
          n169 = call "fgv_cursor_data.vi"("cursor_color_set"=w475, "mode"="Set (Cursor 1 Color)") -> ()  [unwired: 7 in, 7 out]
          n170 = property class="Pnl"(reference=w478, error in=w479) -> ("Decorations[]"=w477:refnum<vi>[])  [unwired: 2 out]
          n171 = Index Array(array=w477, index=1) -> (element=w480:refnum<vi>)
          n172 = property class="Decor"(reference=w480, "BG Color"=w473, "FG Color"=w473) -> ()  [unwired: 1 in, 2 out]
        }
        event "plot_log_phase_vswr": Cursor Move {
          # "Print Cursor Values for Logmag/Phase-Plot"
          n173 = event-data() -> ("CursIdx"=w486:i32, "CursRef"=w487:refnum<vi>)  [unwired: 1 in, 7 out]
          n174 = property on="Property Node" class="Curs"(reference=w487) -> ("Cursor Index"=w485:i32)  [unwired: 1 in, 2 out]
          n175 = local read "plot_log_phase_vswr"() -> (w483:cluster{"array type (2D Dbl)":dbl[], dbl[]}[])
          n176 = call "fgv_cursor_data.vi"("cursor_idx_set"=w486, "plot_data_set"=w483, "cursor_pos_set"=w485, "mode"="Set (Cursor Data)", "plot_id_set"=0) -> ()  [unwired: 4 in, 7 out]
        }
        event "plot_log_phase_vswr": Value Change {
          # "Print Cursor Values for Logmag/Phase-Plot"
          n177 = event-data() -> ("CtlRef"=w489:refnum<vi>, "NewVal"=w491:cluster{"array type (2D Dbl)":dbl[], dbl[]}[])  [unwired: 1 in, 4 out]
          n178 = property on="Property Node" class="XYGraph (strict)"(reference=w489) -> ("CrsrList"=w490:T10)  [unwired: 1 in, 2 out]
          n179 = Array Size(array=w490) -> (size(s)=w492:i32)
          n180 = for {
            N: w492 -> [_]
            tunnel: w490 -> [w506] mode=indexing
            tunnel: w491 -> [w500]
            i -> [w493]
            n181 = Unbundle By Name(w506) -> ("Index"=w494:i32)
            n182 = call "index_one_axis.vi"("x_index"=w494, "curve_sel"=0 ("x_index"), "graph_data"=w500) -> ("Y"=w497:dbl)  [unwired: 7 in, 1 out]
            n183 = call "index_one_axis.vi"("x_index"=w494, "curve_sel"=1 ("x_index"), "graph_data"=w500) -> ("Y"=w498:dbl)  [unwired: 7 in, 1 out]
            n184 = call "index_one_axis.vi"("x_index"=w494, "curve_sel"=2 ("x_index"), "graph_data"=w500) -> ("Y"=w499:dbl, "X"=w496:dbl)  [unwired: 7 in]
            n185 = call "number_with_decimal_points.vi"("Precision"=i16 0, "Double"=w496) -> ("String"=w505:string)  [unwired: 5 in]
            n186 = call "freq_to_wavelength.vi"("frequency_hz"=w496) -> ("wavelength_m"=w495:dbl)  [unwired: 10 in]
            n187 = case shown="0, Default" w493 {
              tunnel: w505 -> [w511 w516]
              tunnel: w498 -> [w510 w513]
              tunnel: w497 -> [w509 w514]
              tunnel: w499 -> [w508 w515]
              tunnel: w495 -> [w507 w512]
              frame 0, Default {
                n188 = local write "cursor_log_phase_freq_1"(w511) -> ()
                n189 = local write "cursor_log_phase_wavel_1"(w507) -> ()
                n190 = local write "cursor_logmag_1"(w509) -> ()
                n191 = local write "cursor_phase_1"(w510) -> ()
                n192 = local write "cursor_vswr_1"(w508) -> ()
              }
              frame 1 {
                n193 = local write "cursor_log_phase_freq_2"(w516) -> ()
                n194 = local write "cursor_log_phase_wavel_2"(w512) -> ()
                n195 = local write "cursor_phase_2"(w513) -> ()
                n196 = local write "cursor_vswr_2"(w515) -> ()
                n197 = local write "cursor_logmag_2"(w514) -> ()
              }
            }
          }
        }
        event "color_picker_logmag": Value Change {
          # "Change Plot Color Logmag/Phase-Plot [Logmag]"
          n198 = event-data() -> ("NewVal"=w517:u32)  [unwired: 1 in, 5 out]
          n199 = property on="plot_log_phase_vswr" class="XYGraph (strict)"("Active Plot"=u32 0, "Plot.Plot Color"=w517) -> ()  [unwired: 2 in, 2 out]
        }
        event "color_picker_phase": Value Change {
          # "Change Plot Color Logmag/Phase-Plot [Phase]"
          n200 = event-data() -> ("NewVal"=w519:u32)  [unwired: 1 in, 5 out]
          n201 = property on="plot_log_phase_vswr" class="XYGraph (strict)"("Active Plot"=u32 1, "Plot.Plot Color"=w519) -> ()  [unwired: 2 in, 2 out]
        }
        event "color_picker_vswr": Value Change {
          # "Change Plot Color Logmag/Phase-Plot [VSWR]"
          n202 = event-data() -> ("NewVal"=w521:u32)  [unwired: 1 in, 5 out]
          n203 = property on="plot_log_phase_vswr" class="XYGraph (strict)"("Active Plot"=u32 2, "Plot.Plot Color"=w521) -> ()  [unwired: 2 in, 2 out]
        }
        event "plot_real_imag": Cursor Move {
          # "Print Cursor Values for Real/Imag-Plot"
          n204 = event-data() -> ("CursIdx"=w526:i32, "CursRef"=w525:refnum<vi>)  [unwired: 1 in, 7 out]
          n205 = property on="Property Node" class="Curs"(reference=w525) -> ("Cursor Index"=w528:i32)  [unwired: 1 in, 2 out]
          n206 = local read "plot_real_imag"() -> (w524:cluster{"array type (2D Dbl)":dbl[], dbl[]}[])
          n207 = call "fgv_cursor_data.vi"("cursor_idx_set"=w526, "plot_data_set"=w524, "cursor_pos_set"=w528, "mode"="Set (Cursor Data)", "plot_id_set"=1) -> ()  [unwired: 4 in, 7 out]
        }
        event "plot_real_imag": Value Change {
          # "Print Cursor Values for Real/Imag-Plot"
          n208 = event-data() -> ("CtlRef"=w532:refnum<vi>, "NewVal"=w533:cluster{"array type (2D Dbl)":dbl[], dbl[]}[])  [unwired: 1 in, 4 out]
          n209 = property on="Property Node" class="XYGraph (strict)"(reference=w532) -> ("CrsrList"=w530:T10)  [unwired: 1 in, 2 out]
          n210 = Array Size(array=w530) -> (size(s)=w531:i32)
          n211 = for {
            N: w531 -> [_]
            tunnel: w533 -> [w542]
            tunnel: w530 -> [w538] mode=indexing
            i -> [w537]
            n212 = Unbundle By Name(w538) -> ("Index"=w536:i32)
            n213 = call "index_two_axes.vi"("x_index"=w536, "graph_data"=w542) -> ("Y2"=w540:dbl, "Y1"=w541:dbl, "X"=w534:dbl)  [unwired: 7 in]
            n214 = call "number_with_decimal_points.vi"("Precision"=i16 0, "Double"=w534) -> ("String"=w539:string)  [unwired: 5 in]
            n215 = call "freq_to_wavelength.vi"("frequency_hz"=w534) -> ("wavelength_m"=w535:dbl)  [unwired: 10 in]
            n216 = case shown="1" w537 {
              tunnel: w541 -> [w547 w548]
              tunnel: w540 -> [w546 w549]
              tunnel: w539 -> [w545 w550]
              tunnel: w535 -> [w544 w551]
              frame 0, Default {
                n217 = local write "cursor_real_1"(w547) -> ()
                n218 = local write "cursor_imag_1"(w546) -> ()
                n219 = local write "cursor_real_imag_freq_1"(w545) -> ()
                n220 = local write "cursor_real_imag_wavel_1"(w544) -> ()
              }
              frame 1 {
                n221 = local write "cursor_real_imag_freq_2"(w550) -> ()
                n222 = local write "cursor_real_imag_wavel_2"(w551) -> ()
                n223 = local write "cursor_real_2"(w548) -> ()
                n224 = local write "cursor_imag_2"(w549) -> ()
              }
            }
          }
        }
        event "color_picker_real": Value Change {
          n225 = event-data() -> ("NewVal"=w552:u32)  [unwired: 1 in, 5 out]
          n226 = property on="plot_real_imag" class="XYGraph (strict)"("Active Plot"=u32 0, "Plot.Plot Color"=w552) -> ()  [unwired: 2 in, 2 out]
        }
        event "color_picker_imag": Value Change {
          n227 = event-data() -> ("NewVal"=w554:u32)  [unwired: 1 in, 5 out]
          n228 = property on="plot_real_imag" class="XYGraph (strict)"("Active Plot"=u32 1, "Plot.Plot Color"=w554) -> ()  [unwired: 2 in, 2 out]
        }
        event "plot_rjx": Cursor Move {
          # "Print Cursor Values for R/jX-Plot"
          n229 = event-data() -> ("CursIdx"=w559:i32, "CursRef"=w558:refnum<vi>)  [unwired: 1 in, 7 out]
          n230 = property on="Property Node" class="Curs"(reference=w558) -> ("Cursor Index"=w557:i32)  [unwired: 1 in, 2 out]
          n231 = call "fgv_cursor_data.vi"("cursor_idx_set"=w559, "cursor_pos_set"=w557, "mode"="Set (Cursor Data)", "plot_id_set"=2) -> ()  [unwired: 5 in, 7 out]
          n232 = local read "plot_rjx"() -> (w572:cluster{"array type (2D Dbl)":dbl[], dbl[]}[])
          n233 = call "index_one_axis.vi"("x_index"=w557, "curve_sel"=0, "graph_data"=w572) -> ("Y"=w561:dbl)  [unwired: 7 in, 1 out]
          n234 = call "index_one_axis.vi"("x_index"=w557, "curve_sel"=1, "graph_data"=w572) -> ("Y"=w562:dbl)  [unwired: 7 in, 1 out]
          n235 = call "index_one_axis.vi"("x_index"=w557, "curve_sel"=2, "graph_data"=w572) -> ("Y"=w563:dbl)  [unwired: 7 in, 1 out]
          n236 = call "index_one_axis.vi"("x_index"=w557, "curve_sel"=3, "graph_data"=w572) -> ("Y"=w564:dbl)  [unwired: 7 in, 1 out]
          n237 = call "index_one_axis.vi"("x_index"=w557, "curve_sel"=4, "graph_data"=w572) -> ("Y"=w565:dbl, "X"=w566:dbl)  [unwired: 7 in]
          n238 = case shown="1" w559 {
            tunnel: w566 -> [w578 w582]
            tunnel: w565 -> [w577 w583]
            tunnel: w564 -> [w576 w584]
            tunnel: w563 -> [w575 w585]
            tunnel: w562 -> [w574 w586]
            tunnel: w561 -> [w573 w587]
            frame 0, Default {
              n239 = local write "cursor_r_1"(w573) -> ()
              n240 = local write "cursor_jx_1"(w574) -> ()
              n241 = local write "cursor_rp_1"(w575) -> ()
              n242 = local write "cursor_jxp_1"(w576) -> ()
              n243 = local write "cursor_z_1"(w577) -> ()
              n244 = call "number_with_decimal_points.vi"("Precision"=i16 0, "Double"=w578) -> ("String"=w579:string)  [unwired: 5 in]
              n245 = call "freq_to_wavelength.vi"("frequency_hz"=w578) -> ("wavelength_m"=w580:dbl)  [unwired: 10 in]
              n246 = local write "cursor_r_jx_freq_1"(w579) -> ()
              n247 = local write "cursor_r_jx_wavel_1"(w580) -> ()
            }
            frame 1 {
              n248 = local write "cursor_r_2"(w587) -> ()
              n249 = local write "cursor_jx_2"(w586) -> ()
              n250 = local write "cursor_rp_2"(w585) -> ()
              n251 = local write "cursor_jxp_2"(w584) -> ()
              n252 = local write "cursor_z_2"(w583) -> ()
              n253 = call "number_with_decimal_points.vi"("Precision"=i16 0, "Double"=w582) -> ("String"=w589:string)  [unwired: 5 in]
              n254 = call "freq_to_wavelength.vi"("frequency_hz"=w582) -> ("wavelength_m"=w590:dbl)  [unwired: 10 in]
              n255 = local write "cursor_r_jx_freq_2"(w589) -> ()
              n256 = local write "cursor_r_jx_wavel_2"(w590) -> ()
            }
          }
        }
        event "plot_rjx": Value Change {
          # "Print Cursor Values for R/jX-Plot"
          n257 = event-data() -> ("CtlRef"=w593:refnum<vi>, "NewVal"=w591:cluster{"array type (2D Dbl)":dbl[], dbl[]}[])  [unwired: 1 in, 4 out]
          n258 = property on="Property Node" class="XYGraph (strict)"(reference=w593) -> ("CrsrList"=w592:T10)  [unwired: 1 in, 2 out]
          n259 = for {
            tunnel: w592 -> [w605] mode=indexing
            tunnel: w591 -> [w601]
            i -> [w604]
            n260 = Unbundle By Name(w605) -> ("Index"=w600:i32)
            n261 = call "index_five_axes.vi"("x_index"=w600, "graph_data"=w601) -> ("Y4"=w595:dbl, "Y3"=w596:dbl, "Y2"=w597:dbl, "Y1"=w598:dbl, "Y5"=w594:dbl, "X"=w599:dbl)  [unwired: 4 in]
            n262 = call "number_with_decimal_points.vi"("Precision"=i16 0, "Double"=w599) -> ("String"=w603:string)  [unwired: 5 in]
            n263 = call "freq_to_wavelength.vi"("frequency_hz"=w599) -> ("wavelength_m"=w602:dbl)  [unwired: 10 in]
            n264 = case shown="1" w604 {
              tunnel: w603 -> [w613 w619]
              tunnel: w597 -> [w610 w617]
              tunnel: w598 -> [w611 w618]
              tunnel: w602 -> [w612 w620]
              tunnel: w596 -> [w609 w616]
              tunnel: w595 -> [w608 w615]
              tunnel: w594 -> [w607 w614]
              frame 0, Default {
                n265 = local write "cursor_r_jx_freq_1"(w613) -> ()
                n266 = local write "cursor_r_jx_wavel_1"(w612) -> ()
                n267 = local write "cursor_r_1"(w611) -> ()
                n268 = local write "cursor_jx_1"(w610) -> ()
                n269 = local write "cursor_rp_1"(w609) -> ()
                n270 = local write "cursor_jxp_1"(w608) -> ()
                n271 = local write "cursor_z_1"(w607) -> ()
              }
              frame 1 {
                n272 = local write "cursor_r_jx_freq_2"(w619) -> ()
                n273 = local write "cursor_r_jx_wavel_2"(w620) -> ()
                n274 = local write "cursor_r_2"(w618) -> ()
                n275 = local write "cursor_jx_2"(w617) -> ()
                n276 = local write "cursor_rp_2"(w616) -> ()
                n277 = local write "cursor_jxp_2"(w615) -> ()
                n278 = local write "cursor_z_2"(w614) -> ()
              }
            }
          }
        }
        event "color_picker_r": Value Change {
          w622 = u32 0 ("Active Plot")
          # "Change Plot Color R/jX-Plot [R]"
          n279 = event-data() -> ("NewVal"=w621:u32)  [unwired: 1 in, 5 out]
          n280 = property on="plot_rjx" class="XYGraph (strict)"("Active Plot"=w622, "Plot.Plot Color"=w621, "ActYScl"=w622, "YScale.ScaleFit"=w622) -> ()  [unwired: 2 in, 2 out]
        }
        event "color_picker_jx": Value Change {
          w625 = u32 1 ("Active Plot")
          # "Change Plot Color R/jX-Plot [jX]"
          n281 = event-data() -> ("NewVal"=w623:u32)  [unwired: 1 in, 5 out]
          n282 = property on="plot_rjx" class="XYGraph (strict)"("Active Plot"=w625, "Plot.Plot Color"=w623, "ActYScl"=w625, "YScale.ScaleFit"=u8 0 ("Y Scale.Scale Fit")) -> ()  [unwired: 2 in, 2 out]
        }
        event "color_picker_rp": Value Change {
          # "Change Plot Color R/jX-Plot [Rp]"
          n283 = event-data() -> ("NewVal"=w626:u32)  [unwired: 1 in, 5 out]
          n284 = property on="plot_rjx" class="XYGraph (strict)"("Active Plot"=u32 2, "Plot.Plot Color"=w626, "ActYScl"=u32 0 ("Active Plot"), "YScale.ScaleFit"=u8 0 ("Y Scale.Scale Fit")) -> ()  [unwired: 2 in, 2 out]
        }
        event "color_picker_jxp": Value Change {
          # "Change Plot Color R/jX-Plot [jXp]"
          n285 = event-data() -> ("NewVal"=w630:u32)  [unwired: 1 in, 5 out]
          n286 = property on="plot_rjx" class="XYGraph (strict)"("Active Plot"=u32 3, "Plot.Plot Color"=w630, "ActYScl"=u32 1 ("Active Plot"), "YScale.ScaleFit"=u8 0 ("Y Scale.Scale Fit")) -> ()  [unwired: 2 in, 2 out]
        }
        event "color_picker_z": Value Change {
          # "Change Plot Color R/jX-Plot [Z]"
          n287 = event-data() -> ("NewVal"=w634:u32)  [unwired: 1 in, 5 out]
          n288 = property on="plot_rjx" class="XYGraph (strict)"("Active Plot"=u32 4, "Plot.Plot Color"=w634, "ActYScl"=u32 0 ("Active Plot"), "YScale.ScaleFit"=u8 0 ("Y Scale.Scale Fit")) -> ()  [unwired: 2 in, 2 out]
        }
        event "plot_lc": Cursor Move {
          w655 = "F" ("unit")
          w654 = "H" ("unit")
          # "Print Cursor Values for R/jX-Plot"
          n289 = event-data() -> ("CursIdx"=w641:i32, "CursRef"=w640:refnum<vi>)  [unwired: 1 in, 7 out]
          n290 = property on="Property Node" class="Curs"(reference=w640) -> ("Cursor Index"=w639:i32)  [unwired: 1 in, 2 out]
          n291 = local read "plot_lc"() -> (w656:cluster{"array type (2D Dbl)":dbl[], dbl[]}[])
          n292 = call "fgv_cursor_data.vi"("cursor_idx_set"=w641, "cursor_pos_set"=w639, "mode"="Set (Cursor Data)", "plot_id_set"=3) -> ()  [unwired: 5 in, 7 out]
          n293 = call "index_four_axes.vi"("x_index"=w639, "graph_data"=w656) -> ("Y4"=w661:dbl, "Y3"=w660:dbl, "Y2"=w658:dbl, "Y1"=w657:dbl, "X"=w659:dbl)  [unwired: 5 in]
          n294 = call "number_with_decimal_points.vi"("Precision"=i16 0, "Double"=w659) -> ("String"=w652:string)  [unwired: 5 in]
          n295 = call "freq_to_wavelength.vi"("frequency_hz"=w659) -> ("wavelength_m"=w651:dbl)  [unwired: 10 in]
          n296 = call "calc_prefix.vi"("unit"=w654, "Numeric in"=w657) -> ("prefix"=w649:string, "Numeric out"=w650:dbl)  [unwired: 8 in]
          n297 = call "calc_prefix.vi"("unit"=w655, "Numeric in"=w658) -> ("prefix"=w647:string, "Numeric out"=w648:dbl)  [unwired: 8 in]
          n298 = call "calc_prefix.vi"("unit"=w654, "Numeric in"=w660) -> ("prefix"=w645:string, "Numeric out"=w646:dbl)  [unwired: 8 in]
          n299 = call "calc_prefix.vi"("unit"=w655, "Numeric in"=w661) -> ("prefix"=w643:string, "Numeric out"=w644:dbl)  [unwired: 8 in]
          n300 = case shown="0, Default" w641 {
            tunnel: w652 -> [w675 w688]
            tunnel: w651 -> [w674 w689]
            tunnel: w650 -> [w673 w690]
            tunnel: w649 -> [w672 w691]
            tunnel: w648 -> [w670 w692]
            tunnel: w647 -> [w669 w693]
            tunnel: w646 -> [w667 w694]
            tunnel: w645 -> [w665 w696]
            tunnel: w644 -> [w664 w695]
            tunnel: w643 -> [w663 w697]
            frame 0, Default {
              n301 = local write "cursor_lc_freq_1"(w675) -> ()
              n302 = local write "cursor_lc_wavel_1"(w674) -> ()
              n303 = local write "cursor_ls_1"(w673) -> ()
              n304 = local write "cursor_ls_1_prefix"(w672) -> ()
              n305 = local write "cursor_cs_1"(w670) -> ()
              n306 = local write "cursor_cs_1_prefix"(w669) -> ()
              n307 = local write "cursor_lp_1"(w667) -> ()
              n308 = local write "cursor_lp_1_prefix"(w665) -> ()
              n309 = local write "cursor_cp_1"(w664) -> ()
              n310 = local write "cursor_cp_1_prefix"(w663) -> ()
              n311 = Less Than 0?(x=w673) -> (x < 0?=w679:bool)
              n312 = Less Than 0?(x=w670) -> (x < 0?=w678:bool)
              n313 = Less Than 0?(x=w667) -> (x < 0?=w677:bool)
              n314 = Less Than 0?(x=w664) -> (x < 0?=w676:bool)
              n315 = case shown="False" w679 {
                tunnel: [u32 6618880 ("Label.BG Color") u32 16711680 ("Label.BG Color")] -> w671
                frame False {
                }
                frame True {
                }
              }
              n316 = case shown="False" w678 {
                tunnel: [u32 6618880 ("Label.BG Color") u32 16711680 ("Label.BG Color")] -> w668
                frame False {
                }
                frame True {
                }
              }
              n317 = case shown="False" w677 {
                tunnel: [u32 6618880 ("Label.BG Color") u32 16711680 ("Label.BG Color")] -> w666
                frame False {
                }
                frame True {
                }
              }
              n318 = case shown="False" w676 {
                tunnel: [u32 6618880 ("Label.BG Color") u32 16711680 ("Label.BG Color")] -> w662
                frame False {
                }
                frame True {
                }
              }
              n319 = property on="cursor_ls_1" class="DigNum (strict)"("NumText.BGColor"=w671) -> ()  [unwired: 2 in, 2 out]
              n320 = property on="cursor_cs_1" class="DigNum (strict)"("NumText.BGColor"=w668) -> ()  [unwired: 2 in, 2 out]
              n321 = property on="cursor_lp_1" class="DigNum (strict)"("NumText.BGColor"=w666) -> ()  [unwired: 2 in, 2 out]
              n322 = property on="cursor_cp_1" class="DigNum (strict)"("NumText.BGColor"=w662) -> ()  [unwired: 2 in, 2 out]
            }
            frame 1 {
              n323 = local write "cursor_lc_freq_2"(w688) -> ()
              n324 = local write "cursor_lc_wavel_2"(w689) -> ()
              n325 = local write "cursor_ls_2"(w690) -> ()
              n326 = local write "cursor_ls_2_prefix"(w691) -> ()
              n327 = local write "cursor_cs_2"(w692) -> ()
              n328 = local write "cursor_cs_2_prefix"(w693) -> ()
              n329 = local write "cursor_lp_2"(w694) -> ()
              n330 = local write "cursor_lp_2_prefix"(w696) -> ()
              n331 = local write "cursor_cp_2"(w695) -> ()
              n332 = local write "cursor_cp_2_prefix"(w697) -> ()
              n333 = Less Than 0?(x=w690) -> (x < 0?=w705:bool)
              n334 = Less Than 0?(x=w692) -> (x < 0?=w704:bool)
              n335 = Less Than 0?(x=w694) -> (x < 0?=w703:bool)
              n336 = Less Than 0?(x=w695) -> (x < 0?=w702:bool)
              n337 = case shown="False" w705 {
                tunnel: [u32 6618880 ("Label.BG Color") u32 16711680 ("Label.BG Color")] -> w701
                frame False {
                }
                frame True {
                }
              }
              n338 = case shown="False" w704 {
                tunnel: [u32 6618880 ("Label.BG Color") u32 16711680 ("Label.BG Color")] -> w700
                frame False {
                }
                frame True {
                }
              }
              n339 = case shown="False" w703 {
                tunnel: [u32 6618880 ("Label.BG Color") u32 16711680 ("Label.BG Color")] -> w699
                frame False {
                }
                frame True {
                }
              }
              n340 = case shown="False" w702 {
                tunnel: [u32 6618880 ("Label.BG Color") u32 16711680 ("Label.BG Color")] -> w698
                frame False {
                }
                frame True {
                }
              }
              n341 = property on="cursor_ls_2" class="DigNum (strict)"("NumText.BGColor"=w701) -> ()  [unwired: 2 in, 2 out]
              n342 = property on="cursor_cs_2" class="DigNum (strict)"("NumText.BGColor"=w700) -> ()  [unwired: 2 in, 2 out]
              n343 = property on="cursor_lp_2" class="DigNum (strict)"("NumText.BGColor"=w699) -> ()  [unwired: 2 in, 2 out]
              n344 = property on="cursor_cp_2" class="DigNum (strict)"("NumText.BGColor"=w698) -> ()  [unwired: 2 in, 2 out]
            }
          }
        }
        event "plot_lc": Value Change {
          n345 = event-data() -> ("CtlRef"=w715:refnum<vi>, "NewVal"=w714:cluster{"array type (2D Dbl)":dbl[], dbl[]}[])  [unwired: 1 in, 4 out]
          n346 = property on="Property Node" class="XYGraph (strict)"(reference=w715) -> ("CrsrList"=w716:T10)  [unwired: 1 in, 2 out]
          n347 = Array Size(array=w716) -> (size(s)=w717:i32)
          n348 = for {
            N: w717 -> [_]
            tunnel: w716 -> [w738] mode=indexing
            tunnel: w714 -> [w737]
            i -> [w728]
            w729 = "H" ("unit")
            w730 = "F" ("unit")
            n349 = Unbundle By Name(w738) -> ("Index"=w736:i32)
            n350 = call "index_four_axes.vi"("x_index"=w736, "graph_data"=w737) -> ("Y4"=w731:dbl, "Y3"=w732:dbl, "Y2"=w733:dbl, "Y1"=w734:dbl, "X"=w735:dbl)  [unwired: 5 in]
            n351 = call "number_with_decimal_points.vi"("Precision"=i16 0, "Double"=w735) -> ("String"=w718:string)  [unwired: 5 in]
            n352 = call "freq_to_wavelength.vi"("frequency_hz"=w735) -> ("wavelength_m"=w719:dbl)  [unwired: 10 in]
            n353 = call "calc_prefix.vi"("unit"=w729, "Numeric in"=w734) -> ("prefix"=w721:string, "Numeric out"=w720:dbl)  [unwired: 8 in]
            n354 = call "calc_prefix.vi"("unit"=w730, "Numeric in"=w733) -> ("prefix"=w723:string, "Numeric out"=w722:dbl)  [unwired: 8 in]
            n355 = call "calc_prefix.vi"("unit"=w729, "Numeric in"=w732) -> ("prefix"=w725:string, "Numeric out"=w724:dbl)  [unwired: 8 in]
            n356 = call "calc_prefix.vi"("unit"=w730, "Numeric in"=w731) -> ("prefix"=w727:string, "Numeric out"=w726:dbl)  [unwired: 8 in]
            n357 = case shown="1" w728 {
              tunnel: w718 -> [w753 w766]
              tunnel: w719 -> [w752 w767]
              tunnel: w720 -> [w751 w768]
              tunnel: w721 -> [w750 w769]
              tunnel: w722 -> [w748 w770]
              tunnel: w723 -> [w747 w771]
              tunnel: w724 -> [w745 w772]
              tunnel: w725 -> [w743 w774]
              tunnel: w726 -> [w742 w773]
              tunnel: w727 -> [w741 w775]
              frame 0, Default {
                n358 = local write "cursor_lc_freq_1"(w753) -> ()
                n359 = local write "cursor_lc_wavel_1"(w752) -> ()
                n360 = local write "cursor_ls_1"(w751) -> ()
                n361 = local write "cursor_ls_1_prefix"(w750) -> ()
                n362 = local write "cursor_cs_1"(w748) -> ()
                n363 = local write "cursor_cs_1_prefix"(w747) -> ()
                n364 = local write "cursor_lp_1"(w745) -> ()
                n365 = local write "cursor_lp_1_prefix"(w743) -> ()
                n366 = local write "cursor_cp_1"(w742) -> ()
                n367 = local write "cursor_cp_1_prefix"(w741) -> ()
                n368 = Less Than 0?(x=w751) -> (x < 0?=w757:bool)
                n369 = Less Than 0?(x=w748) -> (x < 0?=w756:bool)
                n370 = Less Than 0?(x=w745) -> (x < 0?=w755:bool)
                n371 = Less Than 0?(x=w742) -> (x < 0?=w754:bool)
                n372 = case shown="False" w757 {
                  tunnel: [u32 6618880 ("Label.BG Color") u32 16711680 ("Label.BG Color")] -> w749
                  frame False {
                  }
                  frame True {
                  }
                }
                n373 = case shown="False" w756 {
                  tunnel: [u32 6618880 ("Label.BG Color") u32 16711680 ("Label.BG Color")] -> w746
                  frame False {
                  }
                  frame True {
                  }
                }
                n374 = case shown="False" w755 {
                  tunnel: [u32 6618880 ("Label.BG Color") u32 16711680 ("Label.BG Color")] -> w744
                  frame False {
                  }
                  frame True {
                  }
                }
                n375 = case shown="False" w754 {
                  tunnel: [u32 6618880 ("Label.BG Color") u32 16711680 ("Label.BG Color")] -> w740
                  frame False {
                  }
                  frame True {
                  }
                }
                n376 = property on="cursor_ls_1" class="DigNum (strict)"("NumText.BGColor"=w749) -> ()  [unwired: 2 in, 2 out]
                n377 = property on="cursor_cs_1" class="DigNum (strict)"("NumText.BGColor"=w746) -> ()  [unwired: 2 in, 2 out]
                n378 = property on="cursor_lp_1" class="DigNum (strict)"("NumText.BGColor"=w744) -> ()  [unwired: 2 in, 2 out]
                n379 = property on="cursor_cp_1" class="DigNum (strict)"("NumText.BGColor"=w740) -> ()  [unwired: 2 in, 2 out]
              }
              frame 1 {
                n380 = local write "cursor_lc_freq_2"(w766) -> ()
                n381 = local write "cursor_lc_wavel_2"(w767) -> ()
                n382 = local write "cursor_ls_2"(w768) -> ()
                n383 = local write "cursor_ls_2_prefix"(w769) -> ()
                n384 = local write "cursor_cs_2"(w770) -> ()
                n385 = local write "cursor_cs_2_prefix"(w771) -> ()
                n386 = local write "cursor_lp_2"(w772) -> ()
                n387 = local write "cursor_lp_2_prefix"(w774) -> ()
                n388 = local write "cursor_cp_2"(w773) -> ()
                n389 = local write "cursor_cp_2_prefix"(w775) -> ()
                n390 = Less Than 0?(x=w768) -> (x < 0?=w783:bool)
                n391 = Less Than 0?(x=w770) -> (x < 0?=w782:bool)
                n392 = Less Than 0?(x=w772) -> (x < 0?=w781:bool)
                n393 = Less Than 0?(x=w773) -> (x < 0?=w780:bool)
                n394 = case shown="False" w783 {
                  tunnel: [u32 6618880 ("Label.BG Color") u32 16711680 ("Label.BG Color")] -> w779
                  frame False {
                  }
                  frame True {
                  }
                }
                n395 = case shown="False" w782 {
                  tunnel: [u32 6618880 ("Label.BG Color") u32 16711680 ("Label.BG Color")] -> w778
                  frame False {
                  }
                  frame True {
                  }
                }
                n396 = case shown="False" w781 {
                  tunnel: [u32 6618880 ("Label.BG Color") u32 16711680 ("Label.BG Color")] -> w777
                  frame False {
                  }
                  frame True {
                  }
                }
                n397 = case shown="False" w780 {
                  tunnel: [u32 6618880 ("Label.BG Color") u32 16711680 ("Label.BG Color")] -> w776
                  frame False {
                  }
                  frame True {
                  }
                }
                n398 = property on="cursor_ls_2" class="DigNum (strict)"("NumText.BGColor"=w779) -> ()  [unwired: 2 in, 2 out]
                n399 = property on="cursor_cs_2" class="DigNum (strict)"("NumText.BGColor"=w778) -> ()  [unwired: 2 in, 2 out]
                n400 = property on="cursor_lp_2" class="DigNum (strict)"("NumText.BGColor"=w777) -> ()  [unwired: 2 in, 2 out]
                n401 = property on="cursor_cp_2" class="DigNum (strict)"("NumText.BGColor"=w776) -> ()  [unwired: 2 in, 2 out]
              }
            }
          }
        }
        event "plot_smith": Mouse Move {
          w808 = 300 ("top_center")
          # "Print Mouse-Cursor Values for Smith-Plot"
          n402 = event-data() -> ("Coords"=w809:T11)  [unwired: 1 in, 4 out]
          n403 = local read "plot_log_phase_vswr"() -> (w807:cluster{"array type (2D Dbl)":dbl[], dbl[]}[])
          n404 = local read "plot_real_imag"() -> (w804:cluster{"array type (2D Dbl)":dbl[], dbl[]}[])
          n405 = local read "plot_rjx"() -> (w805:cluster{"array type (2D Dbl)":dbl[], dbl[]}[])
          n406 = property on="plot_smith" class="Pict"() -> ("Top"=w793:i32, "Left"=w792:i32)  [unwired: 2 in, 2 out]
          n407 = Insert Into Array(array=w805, new element=w807) -> (w806:cluster{"array type (2D Dbl)":dbl[], dbl[]}[])  [unwired: 1 in]
          n408 = call "get_smith_hover.vi"("smith_pos_left"=w792, "left_center"=w808, "smith_pos_top"=w793, "top_center"=w808, "Coords"=w809, "cursor_data"=w806, "ref_data"=w804) -> ("cursor_pos"=w802:cluster{"r_norm":dbl, "x_norm":dbl}, "cursor_data"=w803:T12)  [unwired: 3 in]
          n409 = Unbundle(w803) -> ("frequency"=w800:dbl, "r"=→"plot_smith_legend_r":dbl, "jx"=→"plot_smith_legend_jx":dbl, "phase"=→"plot_smith_legend_phase":dbl)
          n410 = Unbundle(w802) -> ("r_norm"=→"plot_smith_legend_curs_r":dbl, "x_norm"=→"plot_smith_legend_curs_x":dbl)
          n411 = call "number_with_decimal_points.vi"("Precision"=i16 0, "Double"=w800) -> ("String"=→"plot_smith_legend_freq":string)  [unwired: 5 in]
        }
        event "plot_smith": Mouse Up {
          # "Show separate Smith Plot"
          n412 = event-data() -> ()  [unwired: 1 in, 8 out]
          n413 = property on="show_smith_window" class="Bool (strict)"("Value"=TRUE ("Boolean")) -> ()  [unwired: 2 in, 2 out]
        }
        event "plot_smith": Value Change {
          n414 = event-data() -> ()  [unwired: 1 in, 6 out]
          n415 = property on="plot_log_phase_vswr" class="XYGraph (strict)"() -> ("CrsrList"=w811:T10)  [unwired: 2 in, 2 out]
          n416 = for {
            tunnel: w811 -> [w815] mode=indexing
            i -> [w814]
            n417 = local read "plot_rjx"() -> (w816:cluster{"array type (2D Dbl)":dbl[], dbl[]}[])
            n418 = control-ref of="plot_smith"() -> (w812:refnum<vi>)
            n419 = Unbundle By Name(w815) -> ("Index"=w813:i32)
            n420 = Current VI's Path() -> (path=w817:path)
            n421 = call "set_smith_cursor_plot.vi"("path"=w817, "smith_plot"=w812, "cursor_pos"=w813, "cursor_index"=w814, "plot_rjx"=w816) -> ()  [unwired: 7 in]
          }
        }
        event "sva_cal_file": Value Change {
          n422 = event-data() -> ("NewVal"=w819:string)  [unwired: 1 in, 5 out]
          n423 = call "fgv_sva_mode.vi"("cal_file_in"=w819, "mode"="Set (CAL-File)") -> ()  [unwired: 7 in, 3 out]
        }
        event Timeout {
          n424 = event-data() -> ()  [unwired: 1 in, 3 out]
        }
        event Panel Close? {
          w823 = "Plots" ("section")
          w904 = "Plots" ("section")
          w897 = "Plots" ("section")
          w874 = "Plots" ("section")
          w849 = "Plots" ("section")
          w915 = "Plots" ("section")
          w938 = "Plots" ("section")
          w959 = "Plots" ("section")
          w960 = "Siglent_SSA/SVA" ("section")
          # "Save User Settings"
          n425 = event-data() -> ()  [unwired: 1 in, 4 out]
          n426 = Send Notification(notification=TRUE ("element"), notifier=w980) -> ()  [unwired: 1 in, 2 out]
          n427 = local read "selector_serial_port"() -> (w978:refnum<visa-resource-name>)
          n428 = local read "color_picker_phase"() -> (w958:u32)
          n429 = local read "enable_plot_vswr"() -> (w856:bool)
          n430 = local read "color_picker_jx"() -> (w936:u32)
          n431 = local read "color_picker_cs"() -> (w917:u32)
          n432 = local read "enable_plot_rp"() -> (w876:bool)
          n433 = local read "enable_plot_lp"() -> (w895:bool)
          n434 = call <vilib>:"Application Directory.vi"() -> ("Application Directory"=w840:path)
          n435 = Build Path(base path=w840, name or relative path=path "data/plot_config.ini") -> (appended path=w844:path)
          n436 = call <vilib>:"Open Config Data.vi"("configuration file path"=w844) -> ("error out"=w842:errorcluster, "refnum"=w841:T7)  [unwired: 8 in, 1 out]
          n437 = call-poly <vilib>:"Write Key.vi"("section"="NanoVNA", "error in (no error)"=w842, "value"=w978, "key"="COM_Port", "refnum"=w841) -> ("error out"=w974:errorcluster, "refnum out"=w975:T7)  [unwired: 4 in, 1 out]
          n438 = local read "color_picker_vswr"() -> (w953:u32)
          n439 = local read "color_picker_rp"() -> (w933:u32)
          n440 = local read "color_picker_lp"() -> (w911:u32)
          n441 = local read "enable_plot_real"() -> (w859:bool)
          n442 = local read "enable_plot_jxp"() -> (w879:bool)
          n443 = local read "enable_plot_cp"() -> (w901:bool)
          n444 = local read "sva_ip"() -> (w973:string)
          n445 = call-poly <vilib>:"Write Key.vi"("section"=w960, "error in (no error)"=w974, "value"=w973, "key"="IP_Address", "refnum"=w975) -> ("error out"=w969:errorcluster, "refnum out"=w970:T7)  [unwired: 4 in, 1 out]
          n446 = property on="sva_cal_file" class="CmbBox"() -> ("Strings[]"=w834:string[])  [unwired: 2 in, 2 out]
          n447 = local read "enable_plot_imag"() -> (w862:bool)
          n448 = local read "color_picker_real"() -> (w950:u32)
          n449 = local read "color_picker_jxp"() -> (w928:u32)
          n450 = local read "color_picker_cp"() -> (w908:u32)
          n451 = local read "enable_plot_z"() -> (w884:bool)
          n452 = local read "sva_port"() -> (w972:u16)
          n453 = Array To Spreadsheet String(delimiter (Tab)=";", array=w834, 3:"%s" ("format string")) -> (spreadsheet string=w839:string)
          n454 = local read "color_picker_cursor_1"() -> (w830:u32)
          n455 = call-poly <vilib>:"Write Key.vi"("section"=w960, "error in (no error)"=w969, "value"=w972, "key"="Port", "refnum"=w970) -> ("error out"=w965:errorcluster, "refnum out"=w966:T7)  [unwired: 4 in, 1 out]
          n456 = local read "enable_plot_logmag"() -> (w850:bool)
          n457 = local read "color_picker_imag"() -> (w945:u32)
          n458 = local read "color_picker_z"() -> (w925:u32)
          n459 = local read "enable_plot_ls"() -> (w887:bool)
          n460 = local read "cursor_mode"() -> (w967:bool)
          n461 = local read "enable_plot_r"() -> (w867:bool)
          n462 = local read "color_picker_cursor_2"() -> (w829:u32)
          n463 = call-poly <vilib>:"Write Key.vi"("section"=w959, "error in (no error)"=w965, "value"=w967, "key"="Cursor_Interlock", "refnum"=w966) -> ("error out"=w961:errorcluster, "refnum out"=w962:T7)  [unwired: 4 in, 1 out]
          n464 = local read "color_picker_logmag"() -> (w964:u32)
          n465 = local read "enable_plot_phase"() -> (w853:bool)
          n466 = local read "color_picker_ls"() -> (w920:u32)
          n467 = local read "enable_plot_jx"() -> (w870:bool)
          n468 = local read "enable_plot_cs"() -> (w892:bool)
          n469 = local read "color_picker_r"() -> (w942:u32)
          n470 = call-poly <vilib>:"Write Key.vi"("section"=w959, "error in (no error)"=w961, "value"=w964, "key"="Color_Plot_0_0", "refnum"=w962) -> ("error out"=w955:errorcluster, "refnum out"=w956:T7)  [unwired: 4 in, 1 out]
          n471 = call-poly <vilib>:"Write Key.vi"("section"=w938, "error in (no error)"=w955, "value"=w958, "key"="Color_Plot_0_1", "refnum"=w956) -> ("error out"=w951:errorcluster, "refnum out"=w952:T7)  [unwired: 4 in, 1 out]
          n472 = call-poly <vilib>:"Write Key.vi"("section"=w938, "error in (no error)"=w951, "value"=w953, "key"="Color_Plot_0_2", "refnum"=w952) -> ("error out"=w947:errorcluster, "refnum out"=w948:T7)  [unwired: 4 in, 1 out]
          n473 = call-poly <vilib>:"Write Key.vi"("section"=w938, "error in (no error)"=w947, "value"=w950, "key"="Color_Plot_1_0", "refnum"=w948) -> ("error out"=w943:errorcluster, "refnum out"=w944:T7)  [unwired: 4 in, 1 out]
          n474 = call-poly <vilib>:"Write Key.vi"("section"=w938, "error in (no error)"=w943, "value"=w945, "key"="Color_Plot_1_1", "refnum"=w944) -> ("error out"=w939:errorcluster, "refnum out"=w940:T7)  [unwired: 4 in, 1 out]
          n475 = call-poly <vilib>:"Write Key.vi"("section"=w938, "error in (no error)"=w939, "value"=w942, "key"="Color_Plot_2_0", "refnum"=w940) -> ("error out"=w934:errorcluster, "refnum out"=w935:T7)  [unwired: 4 in, 1 out]
          n476 = call-poly <vilib>:"Write Key.vi"("section"=w915, "error in (no error)"=w934, "value"=w936, "key"="Color_Plot_2_1", "refnum"=w935) -> ("error out"=w930:errorcluster, "refnum out"=w931:T7)  [unwired: 4 in, 1 out]
          n477 = call-poly <vilib>:"Write Key.vi"("section"=w915, "error in (no error)"=w930, "value"=w933, "key"="Color_Plot_2_2", "refnum"=w931) -> ("error out"=w926:errorcluster, "refnum out"=w927:T7)  [unwired: 4 in, 1 out]
          n478 = call-poly <vilib>:"Write Key.vi"("section"=w915, "error in (no error)"=w926, "value"=w928, "key"="Color_Plot_2_3", "refnum"=w927) -> ("error out"=w922:errorcluster, "refnum out"=w923:T7)  [unwired: 4 in, 1 out]
          n479 = call-poly <vilib>:"Write Key.vi"("section"=w915, "error in (no error)"=w922, "value"=w925, "key"="Color_Plot_2_4", "refnum"=w923) -> ("error out"=w918:errorcluster, "refnum out"=w919:T7)  [unwired: 4 in, 1 out]
          n480 = call-poly <vilib>:"Write Key.vi"("section"=w915, "error in (no error)"=w918, "value"=w920, "key"="Color_Plot_3_0", "refnum"=w919) -> ("error out"=w913:errorcluster, "refnum out"=w914:T7)  [unwired: 4 in, 1 out]
          n481 = call-poly <vilib>:"Write Key.vi"("section"=w849, "error in (no error)"=w913, "value"=w917, "key"="Color_Plot_3_1", "refnum"=w914) -> ("error out"=w909:errorcluster, "refnum out"=w910:T7)  [unwired: 4 in, 1 out]
          n482 = call-poly <vilib>:"Write Key.vi"("section"=w849, "error in (no error)"=w909, "value"=w911, "key"="Color_Plot_3_2", "refnum"=w910) -> ("error out"=w905:errorcluster, "refnum out"=w906:T7)  [unwired: 4 in, 1 out]
          n483 = call-poly <vilib>:"Write Key.vi"("section"=w849, "error in (no error)"=w905, "value"=w908, "key"="Color_Plot_3_3", "refnum"=w906) -> ("error out"=w845:errorcluster, "refnum out"=w846:T7)  [unwired: 4 in, 1 out]
          n484 = call-poly <vilib>:"Write Key.vi"("section"=w849, "error in (no error)"=w845, "value"=w850, "key"="Enable_Plot_0_0", "refnum"=w846) -> ("error out"=w855:errorcluster, "refnum out"=w854:T7)  [unwired: 4 in, 1 out]
          n485 = call-poly <vilib>:"Write Key.vi"("section"=w849, "error in (no error)"=w855, "value"=w853, "key"="Enable_Plot_0_1", "refnum"=w854) -> ("error out"=w848:errorcluster, "refnum out"=w847:T7)  [unwired: 4 in, 1 out]
          n486 = call-poly <vilib>:"Write Key.vi"("section"=w874, "error in (no error)"=w848, "value"=w856, "key"="Enable_Plot_0_2", "refnum"=w847) -> ("error out"=w861:errorcluster, "refnum out"=w860:T7)  [unwired: 4 in, 1 out]
          n487 = call-poly <vilib>:"Write Key.vi"("section"=w874, "error in (no error)"=w861, "value"=w859, "key"="Enable_Plot_1_0", "refnum"=w860) -> ("error out"=w865:errorcluster, "refnum out"=w864:T7)  [unwired: 4 in, 1 out]
          n488 = call-poly <vilib>:"Write Key.vi"("section"=w874, "error in (no error)"=w865, "value"=w862, "key"="Enable_Plot_1_1", "refnum"=w864) -> ("error out"=w869:errorcluster, "refnum out"=w868:T7)  [unwired: 4 in, 1 out]
          n489 = call-poly <vilib>:"Write Key.vi"("section"=w874, "error in (no error)"=w869, "value"=w867, "key"="Enable_Plot_2_0", "refnum"=w868) -> ("error out"=w873:errorcluster, "refnum out"=w872:T7)  [unwired: 4 in, 1 out]
          n490 = call-poly <vilib>:"Write Key.vi"("section"=w874, "error in (no error)"=w873, "value"=w870, "key"="Enable_Plot_2_1", "refnum"=w872) -> ("error out"=w878:errorcluster, "refnum out"=w877:T7)  [unwired: 4 in, 1 out]
          n491 = call-poly <vilib>:"Write Key.vi"("section"=w897, "error in (no error)"=w878, "value"=w876, "key"="Enable_Plot_2_2", "refnum"=w877) -> ("error out"=w882:errorcluster, "refnum out"=w881:T7)  [unwired: 4 in, 1 out]
          n492 = call-poly <vilib>:"Write Key.vi"("section"=w897, "error in (no error)"=w882, "value"=w879, "key"="Enable_Plot_2_3", "refnum"=w881) -> ("error out"=w886:errorcluster, "refnum out"=w885:T7)  [unwired: 4 in, 1 out]
          n493 = call-poly <vilib>:"Write Key.vi"("section"=w897, "error in (no error)"=w886, "value"=w884, "key"="Enable_Plot_2_4", "refnum"=w885) -> ("error out"=w890:errorcluster, "refnum out"=w889:T7)  [unwired: 4 in, 1 out]
          n494 = call-poly <vilib>:"Write Key.vi"("section"=w897, "error in (no error)"=w890, "value"=w887, "key"="Enable_Plot_3_0", "refnum"=w889) -> ("error out"=w894:errorcluster, "refnum out"=w893:T7)  [unwired: 4 in, 1 out]
          n495 = call-poly <vilib>:"Write Key.vi"("section"=w897, "error in (no error)"=w894, "value"=w892, "key"="Enable_Plot_3_1", "refnum"=w893) -> ("error out"=w899:errorcluster, "refnum out"=w898:T7)  [unwired: 4 in, 1 out]
          n496 = call-poly <vilib>:"Write Key.vi"("section"=w904, "error in (no error)"=w899, "value"=w895, "key"="Enable_Plot_3_2", "refnum"=w898) -> ("error out"=w903:errorcluster, "refnum out"=w902:T7)  [unwired: 4 in, 1 out]
          n497 = call-poly <vilib>:"Write Key.vi"("section"=w904, "error in (no error)"=w903, "value"=w901, "key"="Enable_Plot_3_3", "refnum"=w902) -> ("error out"=w837:errorcluster, "refnum out"=w838:T7)  [unwired: 4 in, 1 out]
          n498 = call-poly <vilib>:"Write Key.vi"("section"="Siglent_SSA/SVA", "error in (no error)"=w837, "value"=w839, "key"="CAL-File_History", "refnum"=w838) -> ("error out"=w826:errorcluster, "refnum out"=w827:T7)  [unwired: 4 in, 1 out]
          n499 = call-poly <vilib>:"Write Key.vi"("section"=w823, "error in (no error)"=w826, "value"=w830, "key"="Color_Cursor_1", "refnum"=w827) -> ("error out"=w825:errorcluster, "refnum out"=w824:T7)  [unwired: 4 in, 1 out]
          n500 = call-poly <vilib>:"Write Key.vi"("section"=w823, "error in (no error)"=w825, "value"=w829, "key"="Color_Cursor_2", "refnum"=w824) -> ("error out"=w821:errorcluster, "refnum out"=w822:T7)  [unwired: 4 in, 1 out]
          n501 = call <vilib>:"Close Config Data.vi"("error in (no error)"=w821, "refnum"=w822) -> ()  [unwired: 8 in, 2 out]
          n502 = event-data() -> ()  [unwired: 2 in, 1 out]
        }
      }
      n503 = case shown="True" w427 {
        frame False {
        }
        frame True {
          n504 = call "fgv_cursor_data.vi"() -> ("cursor_idx_get"=w449:i32, "cursor_data_get"=w446:T13)  [unwired: 9 in, 5 out]
          n505 = Unbundle(w446) -> ("cursor_data"=w453:dbl[], "frequency"=w448:string, "wavelength_m"=w447:dbl)
          n506 = Index Array(array=w453) -> (element #1=w450:dbl, element #2=w451:dbl, element #3=w452:dbl)  [unwired: 3 in]
          n507 = case shown="0, Default" w449 {
            tunnel: w452 -> [w456 w463]
            tunnel: w451 -> [w455 w462]
            tunnel: w450 -> [w454 w461]
            tunnel: w448 -> [w457 w460]
            tunnel: w447 -> [w458 w459]
            frame 0, Default {
              n508 = local write "cursor_logmag_1"(w454) -> ()
              n509 = local write "cursor_phase_1"(w455) -> ()
              n510 = local write "cursor_vswr_1"(w456) -> ()
              n511 = local write "cursor_log_phase_freq_1"(w457) -> ()
              n512 = local write "cursor_log_phase_wavel_1"(w458) -> ()
            }
            frame 1 {
              n513 = local write "cursor_logmag_2"(w461) -> ()
              n514 = local write "cursor_phase_2"(w462) -> ()
              n515 = local write "cursor_vswr_2"(w463) -> ()
              n516 = local write "cursor_log_phase_freq_2"(w460) -> ()
              n517 = local write "cursor_log_phase_wavel_2"(w459) -> ()
            }
          }
        }
      }
      n518 = case shown="True" w426 {
        frame False {
        }
        frame True {
          n519 = call "fgv_cursor_data.vi"() -> ("cursor_idx_get"=w436:i32, "cursor_data_get"=w431:T13)  [unwired: 9 in, 5 out]
          n520 = Unbundle(w431) -> ("cursor_data"=w437:dbl[], "frequency"=w433:string, "wavelength_m"=w432:dbl)
          n521 = Index Array(array=w437) -> (element #1=w435:dbl, element #2=w434:dbl)  [unwired: 2 in]
          n522 = case shown="0, Default" w436 {
            tunnel: w435 -> [w441 w445]
            tunnel: w434 -> [w440 w444]
            tunnel: w433 -> [w439 w443]
            tunnel: w432 -> [w438 w442]
            frame 0, Default {
              n523 = local write "cursor_real_1"(w441) -> ()
              n524 = local write "cursor_imag_1"(w440) -> ()
              n525 = local write "cursor_real_imag_freq_1"(w439) -> ()
              n526 = local write "cursor_real_imag_wavel_1"(w438) -> ()
            }
            frame 1 {
              n527 = local write "cursor_real_2"(w445) -> ()
              n528 = local write "cursor_imag_2"(w444) -> ()
              n529 = local write "cursor_real_imag_freq_2"(w443) -> ()
              n530 = local write "cursor_real_imag_wavel_2"(w442) -> ()
            }
          }
        }
      }
    }
    n531 = call "Is Value Changed.vim"("value"=w65) -> ("changed or first call?"=w63:bool)
    n532 = call "Is Value Changed.vim"("value"=w50) -> ("changed or first call?"=w61:bool)
    n533 = And(x=w61, y=w50) -> (x .and. y?=w62:bool)
    n534 = Or(x=w63, y=w62) -> (x .or. y?=w64:bool)
    n535 = Or(x=w50, y=w51) -> (x .or. y?=w52:bool)
    n536 = case shown="True" w52 {
      frame False {
        n537 = property on="button_single_sweep" class="Bool"("DisabledEnum"=T3."Disabled and Grayed Out" ("Disabled")) -> ()  [unwired: 2 in, 2 out]
        n538 = property on="button_auto_sweep" class="Bool (strict)"("DisabledEnum"=T3."Disabled and Grayed Out" ("Disabled")) -> ()  [unwired: 2 in, 2 out]
      }
      frame True {
        n539 = property on="button_auto_sweep" class="Bool (strict)"("DisabledEnum"=T3."Enabled" ("Disabled")) -> ("Value"=w182:bool)  [unwired: 2 in, 2 out]
        n540 = case shown="False" w182 {
          tunnel: [T3."Enabled" ("Disabled") T3."Disabled and Grayed Out" ("Disabled")] -> w183
          frame False {
          }
          frame True {
          }
        }
        n541 = property on="button_single_sweep" class="Bool"("DisabledEnum"=w183) -> ()  [unwired: 2 in, 2 out]
      }
    }
    n542 = case shown="True" w51 {
      frame False {
        w414 = T3."Enabled" ("Disabled")
        n543 = property on="selector_serial_port" class="VISAName"("DisabledEnum"=w414) -> ()  [unwired: 2 in, 2 out]
        n544 = property on="button_tcp_connect" class="Bool (strict)"("DisabledEnum"=w414) -> ()  [unwired: 2 in, 2 out]
      }
      frame True {
        w415 = T3."Disabled and Grayed Out" ("Disabled")
        n545 = property on="selector_serial_port" class="VISAName"("DisabledEnum"=w415) -> ()  [unwired: 2 in, 2 out]
        n546 = property on="button_tcp_connect" class="Bool (strict)"("DisabledEnum"=w415) -> ()  [unwired: 2 in, 2 out]
      }
    }
    n547 = case shown="True" w64 {
      tunnel: w65 -> [_ w213]
      frame False {
      }
      frame True {
        n548 = Unbundle(w213) -> ("mode"=w212:string, "s11_s21"=w211:string, "graph"=w210:string, "freq_range"=w204:cluster{"start_freq":string, "stop_freq":string}, "points"=w203:string)
        n549 = case shown="\"VNA\"" w212 {
          tunnel: [T3."Disabled and Grayed Out" ("DisabledEnum") T3."Enabled" ("DisabledEnum")] -> w205
          tunnel: [cluster{u32, u32}[] [{16711680, 16711680}, {4424887, 4424887}, {4424887, 4424887}, {4424887, 4424887}, {4424887, 16777215}, {4424887, 16777215}] ("Colors [4]") cluster{u32, u32}[] [{6618880, 6618880}, {4424887, 4424887}, {4424887, 4424887}, {4424887, 4424887}, {4424887, 16777215}, {4424887, 16777215}] ("Colors [4]")] -> w209
          tunnel: w204 -> [_ w227]
          tunnel: w203 -> [_ w226]
          frame "SA", Default {
          }
          frame "VNA" {
            n550 = call "tcp_sweep_preset.vi"("points_in"=w226, "freq_range"=w227) -> ("points_out"=w223:i32, "stop_freq"=w224:dbl, "start_freq"=w225:dbl)  [unwired: 7 in]
            n551 = local write "sweep_start"(w225) -> ()
            n552 = local write "sweep_stop"(w224) -> ()
            n553 = local write "sweep_points"(w223) -> ()
          }
        }
        n554 = case shown="\"S21\"" w211 {
          tunnel: [w216 cluster{u32, u32}[] [{6618880, 6618880}, {4424887, 4424887}, {4424887, 4424887}, {4424887, 4424887}, {4424887, 16777215}, {4424887, 16777215}] ("Colors [4]") cluster{u32, u32}[] [{11053998, 11053998}, {4424887, 4424887}, {4424887, 4424887}, {4424887, 4424887}, {4424887, 16777215}, {4424887, 16777215}] ("Colors [4]")] -> w208
          tunnel: [w216 cluster{u32, u32}[] [{11053998, 11053998}, {4424887, 4424887}, {4424887, 4424887}, {4424887, 4424887}, {4424887, 16777215}, {4424887, 16777215}] ("Colors [4]") cluster{u32, u32}[] [{6618880, 6618880}, {4424887, 4424887}, {4424887, 4424887}, {4424887, 4424887}, {4424887, 16777215}, {4424887, 16777215}] ("Colors [4]")] -> w207
          frame Default {
            w216 = cluster{u32, u32}[] [{11053998, 11053998}, {4424887, 4424887}, {4424887, 4424887}, {4424887, 4424887}, {4424887, 16777215}, {4424887, 16777215}] ("Colors [4]")
          }
          frame "S11" {
          }
          frame "S21" {
          }
        }
        n555 = case shown="\"SMIT\"" w210 {
          tunnel: [cluster{u32, u32}[] [{16711680, 16711680}, {4424887, 4424887}, {4424887, 4424887}, {4424887, 4424887}, {4424887, 16777215}, {4424887, 16777215}] ("Colors [4]") cluster{u32, u32}[] [{6618880, 6618880}, {4424887, 4424887}, {4424887, 4424887}, {4424887, 4424887}, {4424887, 16777215}, {4424887, 16777215}] ("Colors [4]")] -> w206
          frame "MLOG", Default {
          }
          frame "SMIT" {
          }
        }
        n556 = property on="button_tcp_vna_mode" class="Bool"("Colors [4]"=w209) -> ()  [unwired: 2 in, 2 out]
        n557 = property on="button_tcp_load_cal" class="Bool"("DisabledEnum"=w205) -> ()  [unwired: 2 in, 2 out]
        n558 = property on="button_tcp_s11_mode" class="Bool"("Colors [4]"=w208, "DisabledEnum"=w205) -> ()  [unwired: 2 in, 2 out]
        n559 = property on="button_tcp_s21_mode" class="Bool"("Colors [4]"=w207, "DisabledEnum"=w205) -> ()  [unwired: 2 in, 2 out]
        n560 = property on="button_tcp_smith_mode" class="Bool"("Colors [4]"=w206, "DisabledEnum"=w205) -> ()  [unwired: 2 in, 2 out]
      }
    }
    n561 = case shown="True" "show_smith_window" {
      selector: "show_smith_window" -> [w419 w420]
      tunnel: "show_smith_window" -> [_ w422]
      tunnel: [w419 w421] -> w78
      frame False {
        (unwired) FALSE ("show_smith_window")
      }
      frame True {
        n562 = Open VI Reference(vi path=path "02_ui_smith_plot.vi") -> (vi reference=w424:refnum<vi>)  [unwired: 5 in, 1 out]
        n563 = invoke class="VI" method="FP.Open"(reference=w424, "Activate"=w422, "State"=T4."Standard") -> ()  [unwired: 2 in, 5 out]
        n564 = Not(x=w420) -> (.not. x?=w421:bool)
      }
    }
    n565 = case shown="True" "show_plot_window" {
      tunnel: "show_plot_window" -> [_ w395]
      frame False {
      }
      frame True {
        n566 = Open VI Reference(vi path=path "02_ui_plot_window.vi") -> (vi reference=w397:refnum<vi>)  [unwired: 5 in, 1 out]
        n567 = invoke class="VI" method="FP.Open"(reference=w397, "Activate"=w395, "State"=T4."Standard") -> ()  [unwired: 2 in, 5 out]
      }
    }
    n568 = call "Is Value Changed.vim"("value"="sva_port") -> ("changed or first call?"=w88:bool)
    n569 = call "Is Value Changed.vim"("value"="sva_ip") -> ("changed or first call?"=w87:bool)
    n570 = Or(x=w88, y=w87) -> (x .or. y?=w89:bool)
    n571 = case shown="True" w89 {
      tunnel: "sva_ip" -> [_ w394]
      tunnel: "sva_port" -> [_ w393]
      frame False {
      }
      frame True {
        n572 = call "fgv_tcp_con_param.vi"("mode"="Set (IP/Port)", "port_set"=w393, "ip_address_set"=w394) -> ()  [unwired: 5 in, 4 out]
      }
    }
    n573 = local write "show_smith_window"(w78) -> ()
    n574 = control-ref of="plot_log_phase_vswr"() -> (w114:refnum<vi>)
    n575 = control-ref of="plot_real_imag"() -> (w108:refnum<vi>)
    n576 = call "show_plot.vi"("plot_id"=0 ("y_scale_id"), "show_plot"="enable_plot_logmag", "XYGraph Refnum"=w114) -> ()  [unwired: 8 in, 1 out]
    n577 = call "show_plot.vi"("plot_id"=1 ("y_scale_id"), "show_plot"="enable_plot_phase", "XYGraph Refnum"=w114) -> ()  [unwired: 8 in, 1 out]
    n578 = call "show_plot.vi"("plot_id"=2 ("y_scale_id"), "show_plot"="enable_plot_vswr", "XYGraph Refnum"=w114) -> ()  [unwired: 8 in, 1 out]
    n579 = local read "set_min_vswr_c2"() -> (w26:bool)
    n580 = local read "set_min_vswr_c1"() -> (w29:bool)
    n581 = case shown="True" w29 {
      tunnel: [_ w177] -> w41
      tunnel: [_ 0 ("CursIdx")] -> w40
      tunnel: [w172 99 ("plot_id_get")] -> w38
      tunnel: [_ "Set (Cursor Data)"] -> w27
      frame False {
        n582 = call "fgv_cursor_data.vi"() -> ("plot_id_get"=w172:i32)  [unwired: 9 in, 6 out]
      }
      frame True {
        n583 = local write "set_min_vswr_c1"(FALSE ("set_c1")) -> ()
        n584 = local read "min_vswr_idx"() -> (w177:i32)
      }
    }
    n585 = case shown="True" w26 {
      tunnel: [w165 w169] -> w31
      tunnel: [w166 1 ("CursIdx")] -> w30
      tunnel: w40 -> [w166 _]
      tunnel: w41 -> [w165 _]
      tunnel: [w164 99 ("plot_id_get")] -> w39
      tunnel: w38 -> [w164 _]
      tunnel: w27 -> [w163 _]
      tunnel: [w163 "Set (Cursor Data)"] -> w25
      frame False {
      }
      frame True {
        n586 = local write "set_min_vswr_c2"(FALSE ("set_c1")) -> ()
        n587 = local read "min_vswr_idx"() -> (w169:i32)
      }
    }
    n588 = call "show_plot.vi"("plot_id"=0 ("y_scale_id"), "autoscale"=FALSE, "show_plot"="enable_plot_real", "XYGraph Refnum"=w108) -> ()  [unwired: 7 in, 1 out]
    n589 = call "show_plot.vi"("plot_id"=1 ("y_scale_id"), "autoscale"=FALSE, "show_plot"="enable_plot_imag", "XYGraph Refnum"=w108) -> ()  [unwired: 7 in, 1 out]
    n590 = call "Is Value Changed.vim"("value"="cursor_mode") -> ("changed or first call?"=w35:bool)
    n591 = case shown="True" w35 {
      tunnel: "cursor_mode" -> [_ w139]
      frame False {
      }
      frame True {
        n592 = call "fgv_cursor_data.vi"("cursor_mode_set"=w139, "mode"="Set (Cursor Mode)") -> ()  [unwired: 7 in, 7 out]
      }
    }
    n593 = call "fgv_freq_real_imag.vi"() -> ("plot_data"=w82:T14, "data_array_get"=w83:dbl[][], "freq_array_get"=w81:dbl[])  [unwired: 8 in, 1 out]
    n594 = call "Is Value Changed.vim"("value"=w83) -> ("changed or first call?"=w80:bool)
    n595 = control-ref of="plot_rjx"() -> (w128:refnum<vi>)
    n596 = case shown="True" w80 {
      tunnel: [FALSE TRUE] -> w120
      tunnel: w82 -> [_ w988]
      tunnel: w81 -> [_ w987]
      frame False {
      }
      frame True {
        w1012 = i16 0 ("Precision")
        # "R+jX_Norm"
        # "L/C"
        # "R/jX"
        # "Real/Imag"
        # "Log/Phase/VSWR"
        n597 = Array Subset(array=w988, index=17, length=2) -> (w983:T14)
        n598 = Array Subset(array=w988, index=0, length=3) -> (w999:T14)
        n599 = Array Subset(array=w988, index=3, length=2) -> (w984:T14)
        n600 = Array Subset(array=w988, index=5, length=5) -> (w994:T14)
        n601 = Array Subset(array=w988, index=10, length=4) -> (w991:T14)
        n602 = call "calc_plot_to_smith.vi"("Plot_Data"=w983) -> ("smith plot"=w986:cluster{"r":dbl, "x":dbl}[])  [unwired: 10 in]
        n603 = Array Size(array=w987) -> (size(s)=w1013:i32)
        n604 = Array Max & Min(array=w987) -> (max value=w1010:dbl, min value=w1011:dbl)  [unwired: 2 out]
        n605 = call "prepare_smith_plot.vi"("dimensions (w,h)"=cluster{"width":i16, "height":i16} {"width"=600, "height"=600}, "smith plot"=w986) -> ("smith_out"=w1002:picture)  [unwired: 9 in]
        n606 = local write "points"(w1013) -> ()
        n607 = property on="plot_smith" class="Pict"("Val(Sgnl)"=w1002) -> ()  [unwired: 2 in, 2 out]
        n608 = property on="plot_log_phase_vswr" class="XYGraph (strict)"("Val(Sgnl)"=w999) -> ()  [unwired: 2 in, 2 out]
        n609 = property on="plot_rjx" class="XYGraph (strict)"("Val(Sgnl)"=w994) -> ()  [unwired: 2 in, 2 out]
        n610 = property on="plot_real_imag" class="XYGraph (strict)"("Val(Sgnl)"=w984) -> ()  [unwired: 2 in, 2 out]
        n611 = property on="plot_lc" class="XYGraph (strict)"("Val(Sgnl)"=w991) -> ()  [unwired: 2 in, 2 out]
        n612 = call "number_with_decimal_points.vi"("Precision"=w1012, "Double"=w1010) -> ("String"=w1008:string)  [unwired: 5 in]
        n613 = call "calc_min_vswr.vi"("plot_log_phase_vswr"=w999) -> ("min_vswr_idx"=→"min_vswr_idx":i32, "min_vswr"=w1004:dbl, "min_vswr_freq"=w1007:string)  [unwired: 8 in]
        n614 = call "number_with_decimal_points.vi"("Precision"=w1012, "Double"=w1011) -> ("String"=w1009:string)  [unwired: 5 in]
        n615 = local write "max_frequency"(w1008) -> ()
        n616 = local write "min_frequency"(w1009) -> ()
        n617 = local write "min_vswr_freq"(w1007) -> ()
        n618 = local write "min_vswr"(w1004) -> ()
        n619 = disable-structure shown="Disabled" {
          frame Disabled {
            # "Anpass Linien einzeichnen"
            # "Smith Scale"
            n620 = call <vilib>:"Draw Standard Smith Grid.vi"("Clip Rect"=T5 {"left"=600.0, "top"=0.0, "right"=0.0, "bottom"=600.0}, 9:FALSE ("Show minor"), "Scale Factors"=T6 {"x"={"a"=300.0, "b"=300.0, "log?"=FALSE}, "y"={"a"=-300.0, "b"=300.0, "log?"=FALSE}}) -> ()  [unwired: 8 in, 1 out]
            n621 = call <vilib>:"Draw Smith PolyLine.vi"() -> ()  [unwired: 11 in, 1 out]
          }
          frame Enabled {
          }
        }
        n622 = call "fgv_load_save.vi"() -> ("filename_get"=→"filename":string)  [unwired: 10 in, 1 out]
      }
    }
    n623 = call "set_plot_rjx.vi"("enable_plot_jx"="enable_plot_jx", "set_scale"=w120, "enable_plot_jxp"="enable_plot_jxp", "enable_plot_r"="enable_plot_r", "enable_plot_rp"="enable_plot_rp", "enable_plot_z"="enable_plot_z", "plot_rjx_ref"=w128, "rx_scale_settings"="rx_scale_settings") -> ()  [unwired: 8 in]
    n624 = call "fgv_cursor_data.vi"("cursor_idx_set"=w30, "cursor_pos_set"=w31, "mode"=w25) -> ("cursor_idx_get"=w33:i32, "cursor_pos_get"=w32:i32, "cursor_mode_get"=w36:bool)  [unwired: 6 in, 4 out]
    n625 = call "Is Value Changed.vim"("value"=w32) -> ("changed or first call?"=w28:bool)
    n626 = control-ref of="plot_lc"() -> (w122:refnum<vi>)
    n627 = And(x=w28, y=w36) -> (x .and. y?=w37:bool)
    n628 = call "set_plot_lc.vi"("lc_scale_settings"="lc_scale_settings", "plot_lc_ref"=w122, "set_scale"=w120, "enable_plot_lp"="enable_plot_lp", "enable_plot_ls"="enable_plot_ls", "enable_plot_cp"="enable_plot_cp", "enable_plot_cs"="enable_plot_cs") -> ()  [unwired: 5 in]
    n629 = case shown="True" w37 {
      tunnel: w33 -> [_ w142]
      tunnel: w32 -> [_ w143]
      tunnel: w39 -> [_ w141]
      frame False {
      }
      frame True {
        n630 = local read "plot_rjx"() -> (w144:cluster{"array type (2D Dbl)":dbl[], dbl[]}[])
        n631 = control-ref of="plot_smith"() -> (w145:refnum<vi>)
        n632 = case shown="99, Default" w141 {
          tunnel: w142 -> [_ w162]
          tunnel: w143 -> [_ w161]
          frame 0 {
          }
          frame 99, Default {
            n633 = property on="plot_log_phase_vswr" class="XYGraph (strict)"("Active Cursor"=w162, "Cursor.Cursor Index"=w161) -> (error out=w159:errorcluster, "Value"=w160:cluster{"array type (2D Dbl)":dbl[], dbl[]}[])  [unwired: 2 in, 1 out]
            n634 = property on="plot_log_phase_vswr" class="XYGraph (strict)"(error in=w159, "Val(Sgnl)"=w160) -> ()  [unwired: 1 in, 2 out]
          }
        }
        n635 = case shown="99, Default" w141 {
          tunnel: w142 -> [w158 _]
          tunnel: w143 -> [w157 _]
          frame 99, Default {
            n636 = property on="plot_real_imag" class="XYGraph (strict)"("Active Cursor"=w158, "Cursor.Cursor Index"=w157) -> (error out=w155:errorcluster, "Value"=w156:cluster{"array type (2D Dbl)":dbl[], dbl[]}[])  [unwired: 2 in, 1 out]
            n637 = property on="plot_real_imag" class="XYGraph (strict)"(error in=w155, "Val(Sgnl)"=w156) -> ()  [unwired: 1 in, 2 out]
          }
          frame 1 {
          }
        }
        n638 = case shown="99, Default" w141 {
          tunnel: w142 -> [w154 _]
          tunnel: w143 -> [w153 _]
          frame 99, Default {
            n639 = property on="plot_rjx" class="XYGraph (strict)"("Active Cursor"=w154, "Cursor.Cursor Index"=w153) -> (error out=w151:errorcluster, "Value"=w152:cluster{"array type (2D Dbl)":dbl[], dbl[]}[])  [unwired: 2 in, 1 out]
            n640 = property on="plot_rjx" class="XYGraph (strict)"(error in=w151, "Val(Sgnl)"=w152) -> ()  [unwired: 1 in, 2 out]
          }
          frame 2 {
          }
        }
        n641 = case shown="99, Default" w141 {
          tunnel: w142 -> [w150 _]
          tunnel: w143 -> [w149 _]
          frame 99, Default {
            n642 = property on="plot_lc" class="XYGraph (strict)"("Active Cursor"=w150, "Cursor.Cursor Index"=w149) -> (error out=w147:errorcluster, "Value"=w148:cluster{"array type (2D Dbl)":dbl[], dbl[]}[])  [unwired: 2 in, 1 out]
            n643 = property on="plot_lc" class="XYGraph (strict)"(error in=w147, "Val(Sgnl)"=w148) -> ()  [unwired: 1 in, 2 out]
          }
          frame 3 {
          }
        }
        n644 = Current VI's Path() -> (path=w146:path)
        n645 = call "set_smith_cursor_plot.vi"("path"=w146, "smith_plot"=w145, "cursor_pos"=w143, "cursor_index"=w142, "plot_rjx"=w144) -> ()  [unwired: 7 in]
      }
    }
    n646 = Wait (ms)(milliseconds to wait=u32 15) -> ()  [unwired: 1 out]
  }
  n647 = Release Notifier(notifier=w22) -> ()  [unwired: 2 in, 3 out]
  n648 = Release Notifier(notifier=w13) -> ()  [unwired: 2 in, 3 out]
  n649 = Release Notifier(notifier=w14) -> ()  [unwired: 2 in, 3 out]
  n650 = Release Notifier(notifier=w4) -> ()  [unwired: 2 in, 3 out]
  n651 = Release Notifier(notifier=w21) -> ()  [unwired: 2 in, 3 out]
  n652 = Release Notifier(notifier=w7) -> ()  [unwired: 2 in, 3 out]
  n653 = call "02_get_load_save.vi"() -> ()  [unwired: 12 in]
  n654 = call "02_ui_smith_plot.vi"() -> ()  [unwired: 12 in]
  n655 = call "02_ui_plot_window.vi"() -> ()  [unwired: 12 in]
